vi "MultiPAS-IV.vi"() -> ()   [LabVIEW 2011]
uses:
  <vilib>/Analysis/4window.llb/windowTd.ctl
  sub/QMH/QMH Add Message to Queue (Single Element).vi
  sub/QMH/QMH Add Message to Queue (Array).vi
  <vilib>/measure/maspectr.llb/FFT Spectrum (Mag-Phase) for 1 Chan.vi
  <vilib>/Instr/_visa.llb/VISA Configure Serial Port (Instr).vi
  <vilib>/measure/NI_MAPro.lvlib
  <vilib>/Analysis/NI_AALPro.lvlib
panel:
  out "PAS Save":bool caption="Overtemp"
  in  "Data 2":i32[][](array[numeric])=[[-16374, -7248, 2543, 12030, 20279, 26487, 30037, 30583, 28073, 22744, 15131, 5976, -3818, -13288, -21504, -27663, -31155, -31636, -29064, -23686, -16036, -6862, 2936, 12388, 20571, 26684, 30122, 30546, 27911, 22483, 14793, 5595, -4207, -13644, -21795, -27855, -31232, -31591, -28898, -23423, -15695, -6476, 3323, 12743, 20858, 26873, 30194, 30492, 27744, 22213, 14447, 5207, -4597, -14002, -22082, -28044, -31304, -31540, -28731, -23149, -15348, -6093, 3713, 13101, 21145, 27063, 30265, 30442, 27576, 21943, 14103, 4822, -4984, -14354, -22365, -28230, -31373, -31485, -28556, -22876, -14998, -5702, 4104, 13452, 21428, 27245, 30335, 30388, 27400, 21669, 13754, 4435, -5375, -14705, -22643, -28407, -31436, -31426, -28378, -22598, -14648, -5314, 4497, 13803, 21706, 27423, 30394, 30325, 27221, 21390, 13402, 4045, -5763, -15056, -22921, -28586, -31496, -31361, -28198, -22319, -14297, -4924, 4879, 14151, 21982, 27597, 30451, 30257, 27038, 21107, 13050, 3658, -6149, -15402, -23193, -28754, -31546, -31290, -28010, -22033, -13944, -4536, 5266, 14498, 22252, 27767, 30500, 30184, 26849, 20821, 12696, 3267, -6535, -15748, -23462, -28924, -31596, -31216, -27821, -21748, -13587, -4147, 5653, 14838, 22519, 27930, 30549, 30110, 26658, 20535, 12337, 2878, -6919, -16089, -23727, -29087, -31641, -31137, -27627, -21457, -13229, -3753, 6038, 15181, 22786, 28093, 30591, 30031, 26461, 20243, 11979, 2485, -7303, -16428, -23991, -29244, -31678, -31053, -27426, -21159, -12867, -3360, 6424, 15524, 23043, 28252, 30633, 29946, 26262, 19946, 11617, 2096, -7686, -16764, -24246, -29398, -31712, -30964, -27224, -20862, -12503, -2971, 6803, 15859, 23301, 28401, 30661, 29852, 26058, 19648, 11254, 1703, -8069, -17099, -24500, -29547, -31741, -30870, -27018, -20562, -12138, -2575, 7188, 16192, 23556, 28549, 30689, 29756, 25848, 19348, 10891, 1312, -8448, -17430, -24753, -29691, -31765, -30773, -26806, -20259, -11775, -2186, 7566, 16521, 23801, 28690, 30709, 29656, 25634, 19038, 10523, 919, -8831, -17762, -24997, -29833, -31788, -30672, -26593, -19955, -11409, -1792, 7944, 16850, 24047, 28830, 30724, 29548, 25416, 18729, 10152, 523, -9212, -18092, -25245, -29969, -31805, -30566, -26375, -19647, -11041, -1403, 8319, 17173, 24287, 28963, 30734, 29436, 25192, 18418, 9781, 130, -9587, -18413, -25481, -30101, -31814, -30449, -26150, -19332, -10666, -1007, 8697, 17497, 24524, 29090, 30745, 29325, 24968, 18105, 9408, -263, -9962, -18735, -25718, -30228, -31820, -30334, -25921, -19016, -10296, -618, 9072, 17814, 24756, 29213, 30746, 29202, 24738, 17787, 9036, -657, -10338, -19058, -25951, -30350, -31818, -30214, -25690, -18699, -9922, -224, 9442, 18128, 24984, 29330, 30738, 29078, 24502, 17466, 8658, -1050, -10710, -19371, -26178, -30467, -31814, -30088, -25458, -18382, -9550, 167, 9812, 18440, 25206, 29443, 30732, 28947, 24264, 17143, 8281, -1445, -11083, -19685, -26404, -30581, -31807, -29959, -25221, -18059, -9175, 556, 10178, 18750, 25426, 29548, 30718, 28809, 24018, 16812, 7901, -1842, -11457, -19996, -26624, -30690, -31795, -29824, -24980, -17733, -8799, 950, 10549, 19058, 25643, 29655, 30700, 28673, 23773, 16484, 7523, -2235, -11824, -20304, -26840, -30793, -31772, -29682, -24731, -17402, -8415, 1341, 10916, 19363, 25856, 29755, 30677, 28528, 23522, 16151, 7141, -2626, -12191, -20607, -27051, -30891, -31746, -29536, -24481, -17070, -8035, 1733, 11280, 19664, 26064, 29851, 30648, 28381, 23272, 15818, 6762, -3019, -12555, -20906, -27258, -30984, -31717, -29391, -24226, -16736, -7655, 2128, 11641, 19962, 26270, 29940, 30615, 28229, 23013, 15483, 6376, -3409, -12914, -21204, -27459, -31071, -31684, -29236, -23967, -16398, -7271, 2515, 12005, 20258, 26468, 30024, 30577, 28072, 22753, 15143, 5990, -3802, -13276, -21497, -27660, -31157, -31643, -29076, -23707, -16058, -6886, 2908, 12363, 20550, 26666, 30107, 30536, 27914, 22489, 14805, 5607, -4192, -13633, -21787, -27849, -31230, -31597, -28911, -23438, -15716, -6501, 3298, 12719, 20839, 26858, 30182, 30488, 27744, 22223, 14459, 5225, -4579, -13988, -22071, -28040, -31304, -31549, -28743, -23167, -15368, -6113, 3693, 13076, 21126, 27047, 30255, 30438, 27576, 21950, 14113, 4837, -4971, -14340, -22354, -28224, -31375, -31494, -28570, -22895, -15022, -5725, 4080, 13430, 21408, 27230, 30324, 30384, 27402, 21676, 13766, 4449, -5360, -14694, -22636, -28409, -31440, -31436, -28397, -22617, -14674, -5338, 4467, 13781, 21686, 27408, 30385, 30320, 27224, 21398, 13418, 4062, -5748, -15044, -22913, -28584, -31498, -31368, -28212, -22339, -14321, -4948, 4856, 14131, 21963, 27583, 30440, 30254, 27042, 21118, 13062, 3669, -6137, -15390, -23183, -28751, -31551, -31297, -28024, -22049, -13962, -4556, 5245, 14476, 22235, 27754, 30497, 30186, 26857, 20834, 12710, 3283, -6519, -15733, -23453, -28921, -31600, -31226, -27837, -21765, -13610, -4168, 5628, 14820, 22502, 27918, 30540, 30109, 26664, 20544, 12354, 2891, -6906, -16074, -23719, -29085, -31646, -31148, -27642, -21475, -13251, -3777, 6014, 15160, 22765, 28078, 30583, 30027, 26468, 20251, 11994, 2501, -7292, -16415, -23980, -29242, -31682, -31064, -27443, -21181, -12892, -3386, 6397, 15501, 23026, 28238, 30624, 29944, 26269, 19959, 11633, 2110, -7673, -16753, -24239, -29395, -31719, -30974, -27239, -20882, -12528, -2993, 6782, 15835, 23285, 28390, 30651, 29852, 26063, 19660, 11271, 1720, -8053, -17087, -24493, -29546, -31746, -30880, -27031, -20583, -12163, -2599, 7166, 16173, 23538, 28538, 30684, 29758, 25853, 19356, 10906, 1327, -8433, -17416, -24743, -29688, -31769, -30782, -26821, -20280, -11797, -2208, 7543, 16501, 23786, 28680, 30704, 29656, 25642, 19053, 10540, 936, -8814, -17747, -24989, -29827, -31787, -30678, -26606, -19973, -11430, -1817, 7923, 16829, 24031, 28819, 30721, 29552, 25424, 18746, 10174, 543, -9191, -18072, -25231, -29962, -31802, -30567, -26384, -19660, -11057, -1422, 8302, 17159, 24274, 28952, 30738, 29443, 25205, 18435, 9801, 150, -9568, -18401, -25472, -30095, -31811, -30457, -26163, -19349, -10687, -1031, 8679, 17481, 24511, 29082, 30742, 29327, 24979, 18121, 9431, -241, -9943, -18717, -25707, -30221, -31815, -30337, -25930, -19029, -10312, -631, 9058, 17802, 24745, 29207, 30746, 29209, 24750, 17805, 9057, -634, -10316, -19037, -25937, -30340, -31814, -30217, -25700, -18713, -9939, -240, 9429, 18117, 24976, 29328, 30740, 29088, 24519, 17486, 8682, -1027, -10688, -19352, -26164, -30458, -31810, -30091, -25465, -18390, -9561, 154, 9800, 18433, 25201, 29442, 30735, 28959, 24282, 17165, 8308, -1420, -11063, -19665, -26386, -30570, -31801, -29961, -25227, -18068, -9185, 547, 10171, 18745, 25424, 29552, 30726, 28825, 24038, 16835, 7925, -1815, -11429, -19974, -26608, -30681, -31789, -29826, -24984, -17741, -8807, 938, 10536, 19047, 25636, 29657, 30708, 28685, 23794, 16510, 7550, -2205, -11798, -20280, -26821, -30782, -31766, -29684, -24737, -17411, -8429, 1331, 10906, 19356, 25851, 29758, 30684, 28544, 23546, 16178, 7169, -2598, -12162, -20582, -27035, -30879, -31744, -29540, -24485, -17080, -8048, 1721, 11267, 19655, 26061, 29852, 30654, 28395, 23291, 15843, 6786, -2993, -12527, -20884, -27240, -30974, -31713, -29390, -24230, -16744, -7662, 2115, 11635, 19957, 26268, 29945, 30624, 28246, 23035, 15509, 6406, -3382, -12889, -21180, -27444, -31061, -31677, -29236, -23975, -16408, -7284], [-19329, -1252, 17344, 29341, 30145, 19451, 1353, -17227, -29174, -29920, -19175, -1056, 17506, 29408, 30095, 19300, 1159, -17387, -29238, -29860, -19019, -860, 17671, 29475, 30037, 19143, 960, -17553, -29307, -29809, -18866, -664, 17832, 29545, 29987, 18991, 771, -17707, -29365, -29749, -18707, -466, 17992, 29605, 29926, 18832, 570, -17873, -29434, -29694, -18556, -272, 18151, 29670, 29869, 18676, 375, -18031, -29495, -29633, -18395, -75, 18310, 29729, 29809, 18516, 175, -18194, -29561, -29579, -18238, 120, 18469, 29792, 29750, 18362, -17, -18347, -29617, -29515, -18076, 316, 18629, 29848, 29682, 18197, -218, -18510, -29679, -29456, -17921, 513, 18787, 29910, 29626, 18042, -408, -18664, -29734, -29388, -17757, 709, 18941, 29965, 29560, 17875, -609, -18823, -29791, -29326, -17600, 904, 19095, 30023, 29495, 17717, -802, -18975, -29845, -29260, -17434, 1099, 19251, 30075, 29425, 17551, -1001, -19131, -29901, -29194, -17277, 1296, 19408, 30130, 29359, 17393, -1193, -19284, -29953, -29124, -17112, 1491, 19560, 30184, 29290, 17225, -1392, -19440, -30008, -29056, -16949, 1686, 19713, 30237, 29226, 17069, -1581, -19587, -30054, -28982, -16781, 1883, 19866, 30287, 29151, 16898, -1781, -19742, -30107, -28913, -16616, 2079, 20018, 30337, 29082, 16737, -1973, -19888, -30152, -28838, -16449, 2275, 20167, 30383, 29006, 16564, -2174, -20041, -30200, -28765, -16282, 2471, 20321, 30430, 28934, 16403, -2364, -20187, -30243, -28688, -16113, 2669, 20465, 30470, 28853, 16230, -2568, -20341, -30294, -28618, -15953, 2860, 20615, 30519, 28783, 16070, -2755, -20486, -30335, -28537, -15779, 3057, 20760, 30560, 28700, 15892, -2956, -20637, -30378, -28461, -15613, 3252, 20909, 30605, 28628, 15730, -3145, -20777, -30418, -28377, -15440, 3446, 21054, 30645, 28543, 15557, -3345, -20927, -30460, -28299, -15271, 3643, 21199, 30686, 28465, 15391, -3534, -21066, -30495, -28215, -15100, 3839, 21345, 30722, 28380, 15214, -3734, -21213, -30534, -28134, -14928, 4032, 21487, 30760, 28300, 15044, -3926, -21355, -30570, -28052, -14757, 4225, 21627, 30792, 28209, 14870, -4123, -21501, -30607, -27968, -14586, 4419, 21768, 30832, 28129, 14702, -4314, -21637, -30639, -27880, -14413, 4612, 21907, 30859, 28040, 14521, -4515, -21780, -30675, -27796, -14241, 4804, 22048, 30895, 27953, 14352, -4702, -21919, -30705, -27707, -14064, 4999, 22187, 30922, 27859, 14172, -4900, -22060, -30739, -27620, -13892, 5193, 22326, 30954, 27773, 14003, -5090, -22194, -30765, -27524, -13712, 5386, 22462, 30981, 27679, 13823, -5285, -22333, -30794, -27436, -13538, 5580, 22600, 31013, 27591, 13650, -5476, -22466, -30820, -27343, -13363, 5770, 22732, 31033, 27491, 13468, -5673, -22605, -30848, -27251, -13187, 5964, 22870, 31060, 27401, 13292, -5863, -22736, -30870, -27155, -13010, 6156, 23000, 31079, 27299, 13111, -6058, -22873, -30895, -27060, -12833, 6347, 23134, 31104, 27208, 12936, -6248, -23004, -30918, -26965, -12652, 6536, 23260, 31120, 27106, 12753, -6444, -23136, -30939, -26865, -12472, 6729, 23395, 31148, 27011, 12578, -6634, -23266, -30959, -26766, -12296, 6919, 23523, 31161, 26907, 12392, -6830, -23402, -30982, -26665, -12115, 7109, 23652, 31180, 26809, 12213, -7016, -23524, -30992, -26564, -11932, 7301, 23777, 31195, 26704, 12032, -7210, -23655, -31011, -26464, -11755, 7492, 23907, 31211, 26605, 11855, -7395, -23778, -31024, -26358, -11573, 7680, 24031, 31218, 26494, 11665, -7592, -23908, -31039, -26258, -11392, 7871, 24158, 31237, 26394, 11491, -7775, -24031, -31050, -26153, -11210, 8063, 24281, 31247, 26285, 11302, -7972, -24159, -31062, -26046, -11027, 8250, 24407, 31258, 26180, 11124, -8157, -24276, -31067, -25937, -10841, 8438, 24526, 31265, 26071, 10936, -8347, -24401, -31078, -25829, -10659, 8630, 24649, 31275, 25965, 10755, -8533, -24522, -31087, -25721, -10474, 8816, 24770, 31280, 25853, 10566, -8726, -24641, -31091, -25608, -10290, 9003, 24891, 31287, 25746, 10386, -8910, -24756, -31095, -25498, -10105, 9192, 25008, 31287, 25627, 10196, -9102, -24881, -31101, -25386, -9919, 9381, 25127, 31296, 25521, 10019, -9284, -24994, -31099, -25268, -9732, 9570, 25243, 31293, 25403, 9826, -9476, -25113, -31105, -25157, -9544, 9756, 25359, 31298, 25291, 9645, -9655, -25225, -31099, -25040, -9359, 9942, 25473, 31291, 25167, 9453, -9847, -25341, -31102, -24926, -9173, 10124, 25586, 31294, 25057, 9269, -10029, -25450, -31095, -24809, -8986, 10310, 25696, 31284, 24931, 9078, -10218, -25564, -31094, -24688, -8798, 10497, 25812, 31287, 24819, 8896, -10399, -25673, -31085, -24567, -8608, 10682, 25922, 31278, 24698, 8703, -10587, -25785, -31080, -24448, -8422, 10866, 26033, 31274, 24582, 8522, -10765, -25890, -31067, -24321, -8230, 11050, 26140, 31263, 24455, 8325, -10952, -26001, -31064, -24201, -8040, 11234, 26248, 31255, 24338, 8142, -11132, -26106, -31054, -24079, -7852, 11417, 26353, 31243, 24207, 7948, -11316, -26217, -31041, -23952, -7662, 11601, 26464, 31236, 24089, 7763, -11494, -26315, -31025, -23829, -7471, 11782, 26562, 31217, 23957, 7567, -11682, -26422, -31014, -23702, -7282, 11962, 26667, 31205, 23834, 7383, -11859, -26521, -30998, -23575, -7092, 12144, 26770, 31187, 23704, 7186, -12043, -26626, -30981, -23444, -6900, 12328, 26875, 31176, 23582, 7003, -12218, -26724, -30962, -23316, -6709, 12505, 26971, 31154, 23446, 6805, -12401, -26825, -30946, -23189, -6517, 12687, 27073, 31139, 23322, 6620, -12576, -26919, -30922, -23054, -6323, 12867, 27170, 31114, 23185, 6422, -12760, -27022, -30904, -22923, -6132, 13047, 27272, 31096, 23060, 6237, -12934, -27114, -30879, -22790, -5940, 13222, 27362, 31068, 22921, 6041, -13116, -27212, -30855, -22657, -5748, 13401, 27461, 31048, 22790, 5853, -13289, -27302, -30828, -22522, -5555, 13577, 27549, 31019, 22652, 5652, -13472, -27398, -30806, -22388, -5362, 13753, 27645, 30995, 22521, 5463, -13642, -27487, -30776, -22248, -5169, 13928, 27733, 30963, 22376, 5266, -13823, -27584, -30750, -22113, -4975, 14106, 27828, 30937, 22246, 5082, -13992, -27669, -30717, -21974, -4782, 14280, 27914, 30902, 22101, 4880, -14174, -27760, -30689, -21837, -4588, 14454, 28006, 30875, 21965, 4692, -14340, -27843, -30653, -21693, -4391, 14631, 28092, 30840, 21822, 4494, -14519, -27934, -30620, -21552, -4198, 14805, 28179, 30808, 21688, 4308, -14687, -28015, -30582, -21410, -4004, 14975, 28262, 30770, 21540, 4106, -14861, -28103, -30548, -21268, -3808, 15149, 28349, 30739, 21402, 3916, -15032, -28183, -30512, -21124, -3614, 15319, 28430, 30697, 21255, 3715, -15205, -28267, -30475, -20982, -3421, 15490, 28513, 30664, 21116, 3524, -15376, -28348, -30435, -20837, -3225, 15660, 28592, 30617, 20962, 3327, -15550, -28432, -30397, -20695, -3032, 15829, 28673, 30581, 20820, 3134, -15711, -28506, -30353, -20546, -2837, 15994, 28746, 30530, 20669, 2933, -15887, -28585, -30311, -20400, -2641, 16167, 28828, 30496, 20528, 2745, -16052, -28660, -30264, -20248, -2445, 16335, 28901, 30445, 20376, 2544, -16221, -28737, -30219, -20102, -2250, 16505, 28983, 30406, 20231, 2357, -16381, -28808, -30171, -19950, -2053, 16670, 29053, 30355, 20075, 2154, -16552, -28883, -30127, -19803, -1859, 16835, 29128, 30308, 19930, 1965, -16714, -28952, -30073, -19650, -1663, 17001, 29192, 30255, 19772, 1764, -16881, -29028, -30026, -19496, -1467, 17165, 29268, 30208, 19626, 1572, -17043, -29095, -29977, -19346]]
  out "Filtering":bool caption="Time has Elapsed"
  in  "Switch Filter":bool
  in  "Auto Filter":bool
  out "Elapsed Time (min)":dbl caption="Elapsed Time (s)" format="%#.1g"
  in  "Filter Length (min)":dbl=6.0 caption="Time Target (s)"
  in  "Sample Length (min)":dbl=24.0 caption="Time Target (s)" format="%#.1f"
  out "Time has Elapsed":bool
  in  "Time Target (s)":dbl=1.0
  out "PD Save":bool caption="Overtemp"
  in  "sweep":bool
  in  "All Emit":bool
  in  "Alignment Mode":bool
  in  "660 Emission":bool
  in  "660 Power (mW)":dbl(slide)=100.0 min=0.0 max=100.0 step=1.0 scale=0.0..100.0
  in  "532 Emission":bool
  in  "532 Power (mW)":dbl(slide)=80.0 min=0.0 max=80.0 step=1.0 scale=0.0..80.0
  in  "405 Power (mW)":dbl(slide)=100.0 min=0.0 max=100.0 step=1.0 scale=0.0..100.0
  in  "405 Emission":bool
  out "Overtemp":bool
  in  "Tab Control":T1(tab)=enum."Frequency Sweep"
  in  "Calibration Filepath":path
  in  "Save Cal?":bool=TRUE
  in  "pd id":u32=1
  in  "mic id":u32
  in  "mic cal, scu":dbl=5.41531278804282e-05 format="%#_3e"
  in  "mic cal, scu":dbl=5.59307241877627e-05 format="%#_3e"
  in  "405 Port":refnum<visa-resource-name>="COM70"
  in  "532 Port":refnum<visa-resource-name>="COM26"
  in  "660 Port":refnum<visa-resource-name>="COM69"
  in  "Teensy Port":refnum<visa-resource-name>="COM61"
  in  "Save Mic?":bool
  in  "Mic Time Series File Path":path
  out "error out":errorcluster
  in  "PD Time Series File Path":path
  in  "Save PD?":bool
  in  "Frequency Sweep File Path":path
  in  "Save sweeps?":bool
  in  "Save Abs?":bool
  in  "Abs Time Series File Path":path
  in  "check freqs?":bool=TRUE
  in  "autosweep":bool=TRUE
  in  "set freqs":bool
  out "Frequency Scan":cluster{i32[], "Best Gaussian Fit":dbl[]}[](graph)
  out "Calculated Resonance (Hz)":dbl=1370.0
  in  "Data Start Frequency (Hz)":i32=1355
  in  "Data End Frequency (Hz)":i32=1385
  out "Step No.":i32
  in  "405 F (Hz)":i32=1368
  in  "532 F (Hz)":i32=1372
  in  "660 F (Hz)":i32=1370
  in  "sweep?":bool=TRUE
  in  "660 PD Cal 3":dbl=0.793
  in  "532 PD Cal 3":dbl=0.454
  in  "405 PD Cal 3":dbl=0.237
  out "PD Waveform":waveform(i32)(graph)
  out "PD FFT":cluster{"f0":dbl, "df":dbl, "magnitude":dbl[]}(graph)
  out "pd ts":cluster{dbl, dbl, dbl}(graph)
  in  "Chart Rolling Average Number\n(Transfers to Absorption Data!)":i32=1
  out "mic ts":cluster{dbl, dbl, dbl}(graph)
  out "Mic FFT":cluster{"f0":dbl, "df":dbl, "magnitude":dbl[]}(graph)
  out "Mic Waveform":waveform(i32)(graph)
  in  "calibrate":bool
  in  "GO3 Filepath":path=path "S:/Groups/Smith_G/Photoacoutic Spectroscopy/calibrations/20160810_cal_go3.txt"
  in  "Photodiode Filepath":path=path "S:/Groups/Smith_G/Photoacoutic Spectroscopy/calibrations/20160810_cal_pd.txt"
  in  "Microphone Filepath":path=path "S:/Groups/Smith_G/Photoacoutic Spectroscopy/calibrations/20160810_cal_mic.txt"
  in  "Bkg Start Index":i32=5
  out "aligned data":cluster{"Array":i32[], dbl[]}[](graph)
  out "Calibration":cluster{dbl[], dbl[]}[](graph)
  in  "Bkg End Index":i32=15
  in  "O3 Flow, sccm (80)":dbl=80.0
  in  "660 PD Cal":dbl=0.793
  in  "532 PD Cal":dbl=0.454
  out "532 Slope":dbl
  out "660 Slope":dbl
  out "PAS Cal Coefficient":dbl format="%0.2f"
  in  "GO3 Offset":i32=15
  in  "Cell Calibration, mV/mW":dbl=600000.0
  in  "getbkg":bool
  out "AAE":dbl(graph)
  in  "Bkg Values (mV)":cluster{dbl, dbl, dbl}
  out "Absorption Spectrum":cluster{dbl[], "Best Power Fit":dbl[]}[](graph)
  out "abs ts":cluster{dbl, dbl, dbl}(graph)
  out "Temperatures":T2
  out "Status":string
  in  "Exit":bool
  in  "State Variables":cluster{"CurrentFile":path}
  # "MultiPAS-RGB | AeroSmith Labs (2016)"
  # "Laser Control"
  # "Filter Control"
  # "Communications"
  # "Sound Card Parameters"
  # "Readout"
  # "PD Calibration"
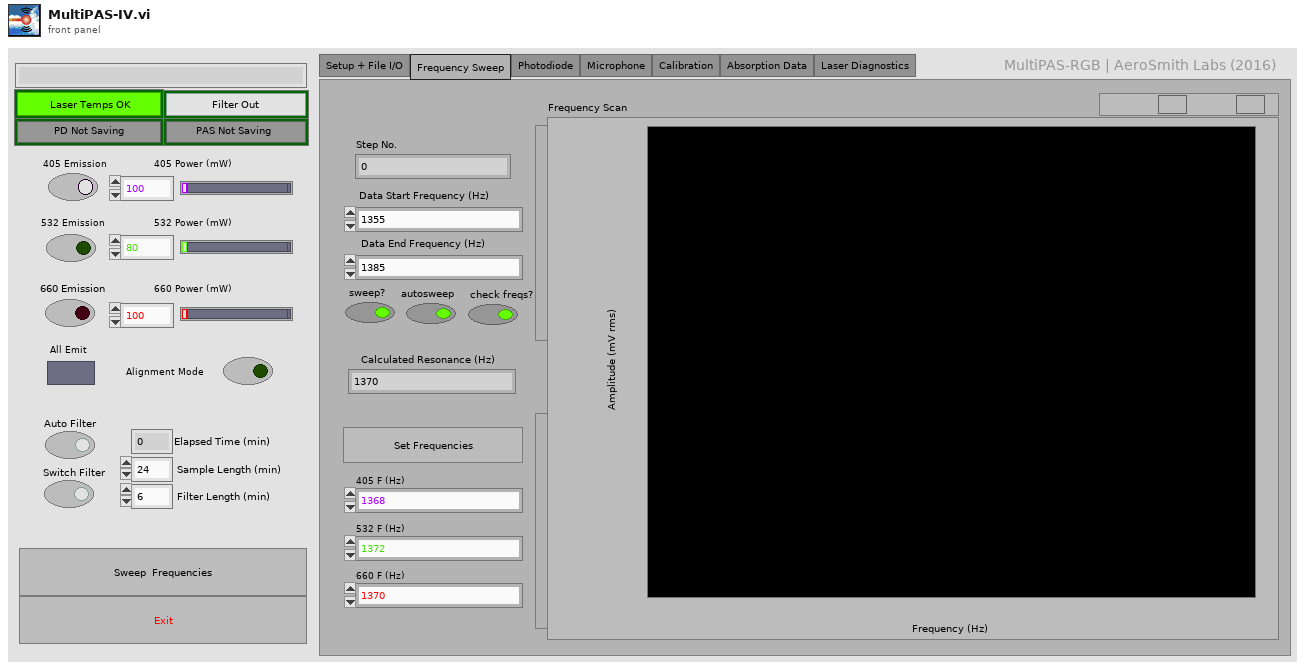
[diagram p1: front panel]
types:
  T1 = enum32{"Setup + File I/O", "Frequency Sweep", "Photodiode", "Microphone", "Calibration", "Absorption Data", "Laser Diagnostics"}
  T2 = cluster{" 405 Temp (C)":dbl, "532 Temp (C)":dbl, "660 Temp (C)":dbl}
  T3 = cluster{"# buffers":i32, "Buffer size":i32, "unit (ms)":enum16{"time (ms)", "Samples"}}
  T4 = typedef "SoundHandle.ctl" = cluster{"DeviceID":u16, "Samples/buf":u32, "Sampl rate":u32, "Bits/sample":u16, "Channels":u8, "Opened":bool}
  T5 = typedef "NI_AALPro.lvlib/windowTd.ctl" = u32
  T6 = cluster{"660 New Array":dbl[], "660 Mean":dbl, "660 SD":dbl}
  T7 = cluster{"532 New Array":dbl[], "532 Mean":dbl, "532 SD":dbl}
  T8 = cluster{"405 New Array":dbl[], "405 Mean":dbl, "405 SD":dbl}
  T9 = cluster{"405 Mean":dbl, "532 Mean":dbl, "660 Mean":dbl}
  T10 = cluster{"Temp (C)":dbl, "Temp (C)":dbl, "Temp (C)":dbl}
  T11 = typedef "LVCursorListTypeDef.ctl" = cluster{"Name":string, "Color":u32, "Style":u8, "Point Style":u8, "Name Visible":bool, "Allow Drag":bool, "Cursor Mode":u32, "Plot":i32, "Index":i32, "Position":cluster{"X":dbl, "Y":dbl}, "X Scale":u32, "Y Scale":u32, "Watch Plots":i32[], "Watch All Plots":bool, "Plot Area":i32, "Label Offset":cluster{"X":dbl, "Y":dbl}}[]
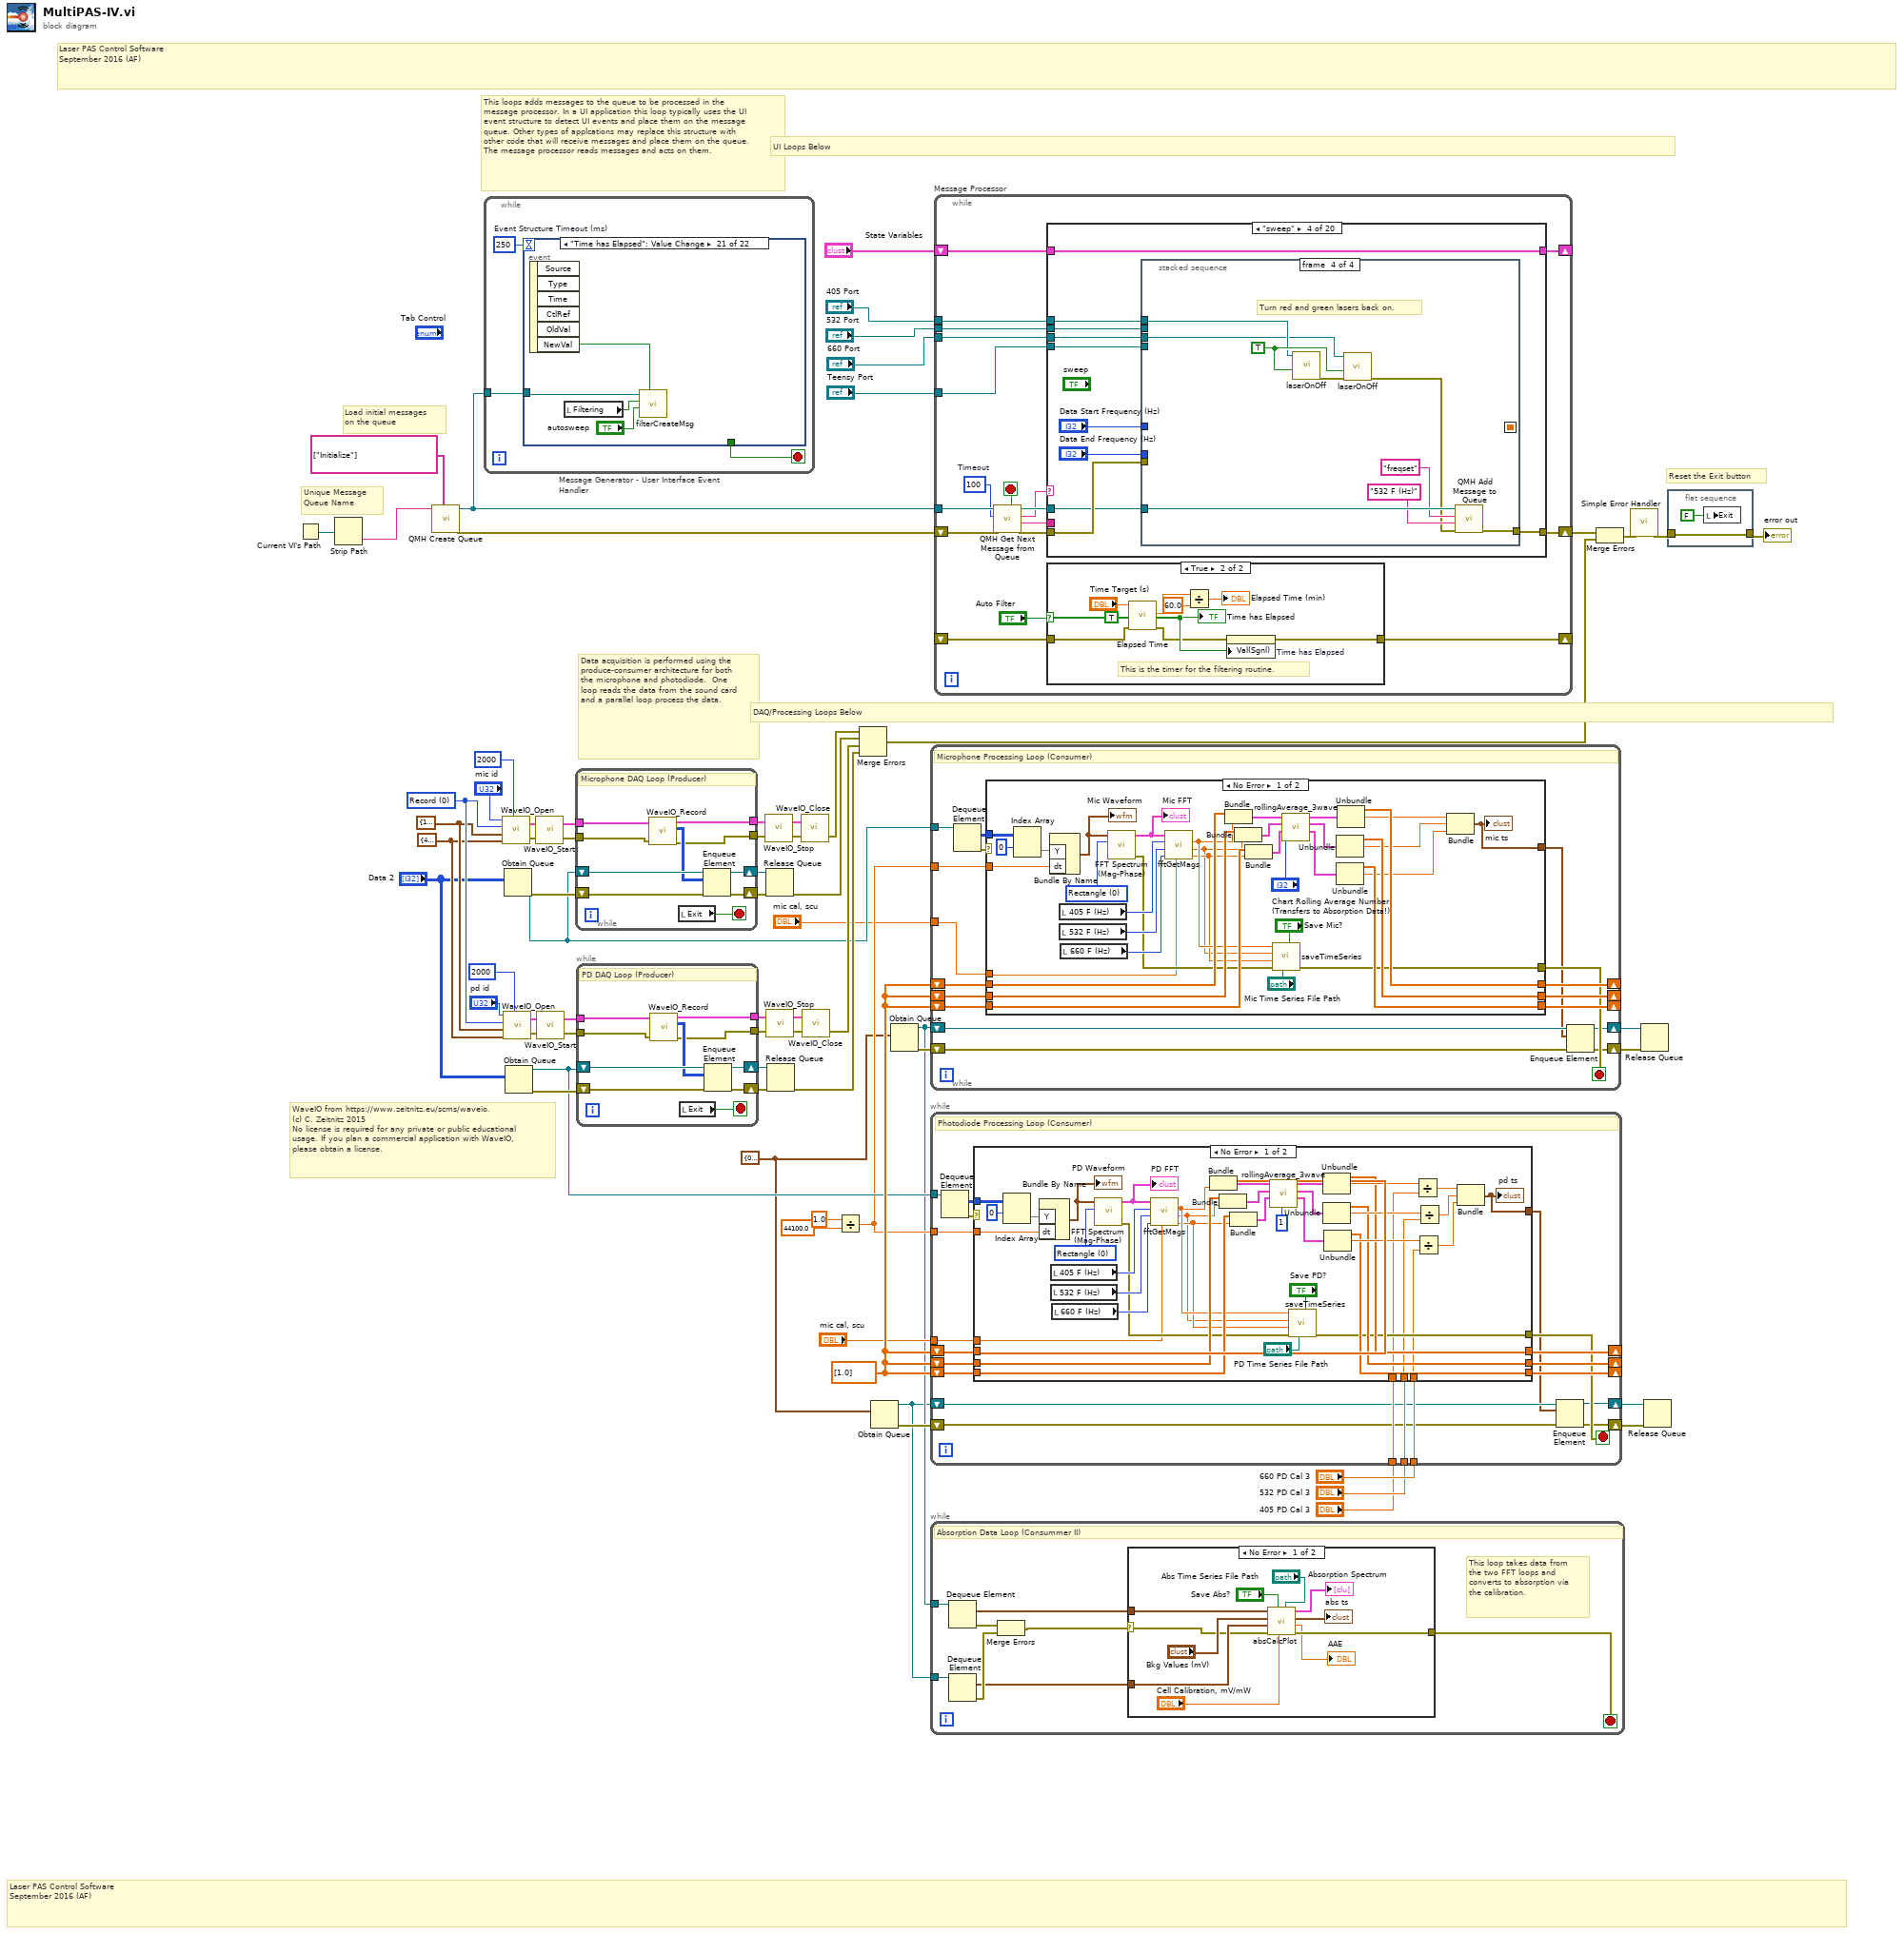
[diagram p0: block diagram]
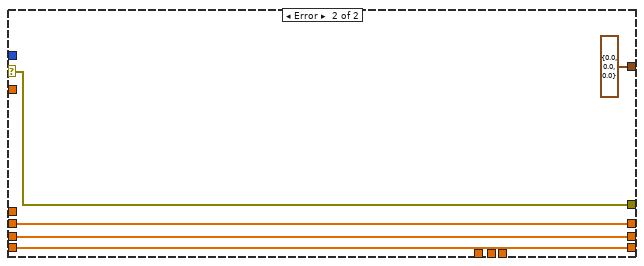
[diagram p3: hidden frame]
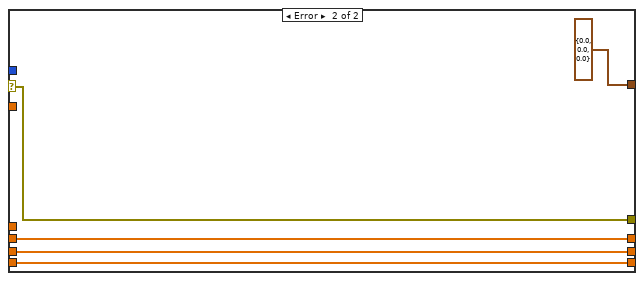
[diagram p4: hidden frame]
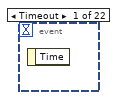
[diagram p5: hidden frame]
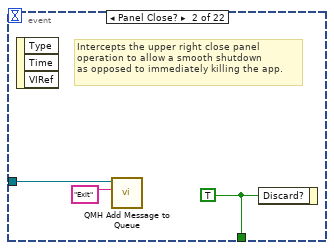
[diagram p6: hidden frame]
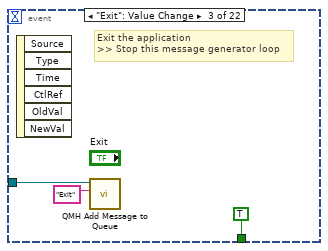
[diagram p7: hidden frame]
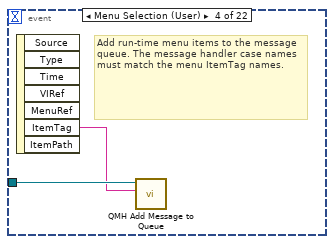
[diagram p8: hidden frame]
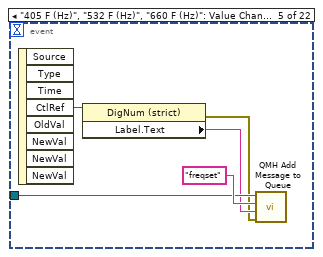
[diagram p9: hidden frame]
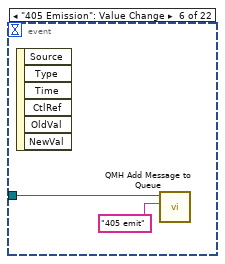
[diagram p10: hidden frame]
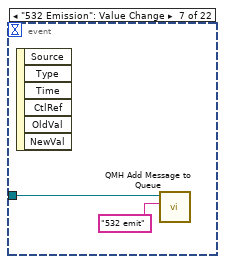
[diagram p11: hidden frame]
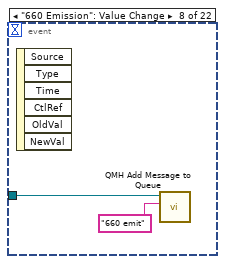
[diagram p12: hidden frame]
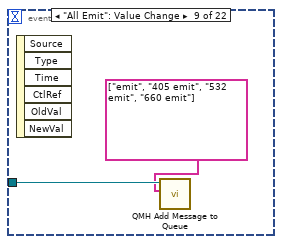
[diagram p13: hidden frame]
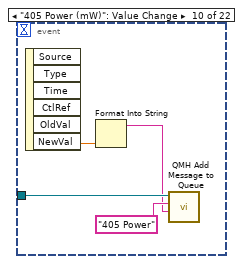
[diagram p14: hidden frame]
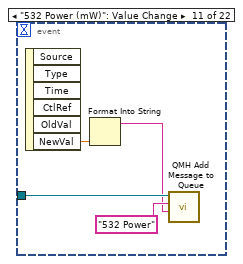
[diagram p15: hidden frame]
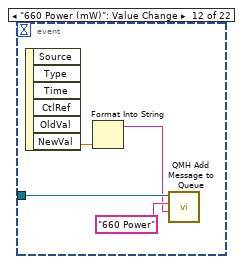
[diagram p16: hidden frame]
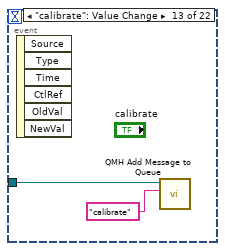
[diagram p17: hidden frame]
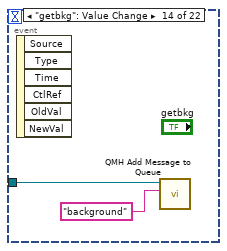
[diagram p18: hidden frame]
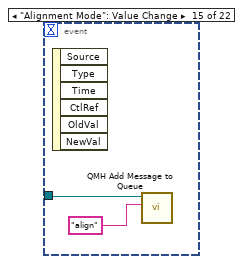
[diagram p19: hidden frame]
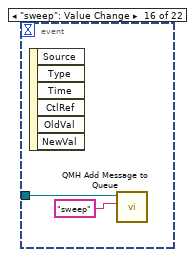
[diagram p20: hidden frame]
diagram:
  w22 = T3 {"# buffers"=10, "Buffer size"=44100, "unit (ms)"=enum."Samples"} ("Buffer")
  w21 = cluster{"Rate":i32, "Bits":i32, "Channels":i32} {"Rate"=44100, "Bits"=24, "Channels"=2} ("Format")
  w1 = cluster{dbl, dbl, dbl} {0.0, 0.0, 0.0}
  w23 = u16 0 items=["Record", "Play", "Loopback", "ASIO input", "ASIO output"] ("Direction (Record)")
  w53 = dbl[] [1.0] ("X")
  # "Laser PAS Control Software\nSeptember 2016 (AF)"
  # "Laser PAS Control Software\nSeptember 2016 (AF)"
  # "Data acquisition is performed using the produce-consumer architecture for both the microphone and photodiode.  One loop reads the data from the sound card and a parallel loop process the data."
  # "WaveIO from https://www.zeitnitz.eu/scms/waveio.\n(c) C. Zeitnitz 2015\nNo license is required for any private or public educational usage. If you plan a commercial application with WaveIO, please obtain a license."
  # "This loops adds messages to the queue to be processed in the message processor. In a UI application this loop typically uses the UI event structure to detect UI events and place them on the message queue. Other types of applcations may replace this structure with other code that will receive messages and place them on the queue.  The message processor reads messages and acts on them."
  # "Reset the Exit button"
  # "Unique Message\nQueue Name"
  # "Load initial messages\non the queue"
  # "DAQ/Processing Loops Below"
  # "UI Loops Below"
  n1 = Current VI's Path() -> (path=w68:path)
  n2 = Strip Path(path=w68) -> (name=w69:string)  [unwired: 1 out]
  n3 = call "QMH Create Queue.vi"("Initial Messages"=string[] ["Initialize"], "Message queue name (unnamed)"=w69) -> ("error out"=w65:errorcluster, "queue out"=w50:refnum<queue>)  [unwired: 8 in]
  n4 = while "Message Generator - User Interface Event Handler" {
    tunnel: w50 -> [w70]
    stop <- w71 stop-if-true
    w72 = 250  # Event Structure Timeout (ms)
    n5 = event shown="[20] \"Time has Elapsed\": Value Change" {
      selector: _ -> [_ _ _ _ _ _ _ _ _ _ _ _ _ _ _ _ _ _ _ _ _ _]
      dyn-events: _ -> [_ _ _ _ _ _ _ _ _ _ _ _ _ _ _ _ _ _ _ _ _ _]
      timeout: w72 -> [_ _ _ _ _ _ _ _ _ _ _ _ _ _ _ _ _ _ _ _ _ _]
      tunnel: [_ w75 TRUE ("Discard?") _ _ _ _ _ _ _ _ _ _ _ _ _ _ _ _ _ _ _] -> w71
      tunnel: w70 -> [_ w74 w77 w80 w84 w86 w88 w90 w93 w96 w100 w104 w106 w108 w110 w113 w117 _ _ w124 w128 w133]
      event Timeout {
        n6 = event-data() -> ()  [unwired: 1 in, 1 out]
      }
      event Panel Close? {
        w75 = TRUE ("Discard?")
        # "Intercepts the upper right close panel\noperation to allow a smooth shutdown\nas opposed to immediately killing the app."
        n7 = event-data() -> ()  [unwired: 1 in, 3 out]
        n8 = call-poly "QMH Add Message to Queue.vi"("Message"="Exit", "queue in"=w74) -> ()  [unwired: 8 in, 2 out]
        n9 = event-data("Discard?"=w75) -> ()  [unwired: 1 in, 1 out]
      }
      event "Exit": Value Change {
        # "Exit the application\n>> Stop this message generator loop"
        n10 = event-data() -> ()  [unwired: 1 in, 6 out]
        n11 = call-poly "QMH Add Message to Queue.vi"("Message"="Exit", "queue in"=w77) -> ()  [unwired: 8 in, 2 out]
      }
      event Menu Selection (User) {
        # "Add run-time menu items to the message\nqueue. The message handler case names must match the menu ItemTag names."
        n12 = event-data() -> ("ItemTag"=w79:string)  [unwired: 1 in, 6 out]
        n13 = call-poly "QMH Add Message to Queue.vi"("Message"=w79, "queue in"=w80) -> ()  [unwired: 8 in, 2 out]
      }
      event "405 F (Hz)", "532 F (Hz)", "660 F (Hz)": Value Change {
        n14 = event-data() -> ("CtlRef"=w83:refnum<vi>)  [unwired: 1 in, 7 out]
        n15 = property class="DigNum (strict)"(reference=w83) -> (error out=w81:errorcluster, "Label.Text"=w82:string)  [unwired: 1 in, 1 out]
        n16 = call-poly "QMH Add Message to Queue.vi"("error in (no error)"=w81, "Parameter"=w82, "Message"="freqset", "queue in"=w84) -> ()  [unwired: 6 in, 2 out]
      }
      event "405 Emission": Value Change {
        n17 = event-data() -> ()  [unwired: 1 in, 6 out]
        n18 = call-poly "QMH Add Message to Queue.vi"("Message"="405 emit", "queue in"=w86) -> ()  [unwired: 8 in, 2 out]
      }
      event "532 Emission": Value Change {
        n19 = event-data() -> ()  [unwired: 1 in, 6 out]
        n20 = call-poly "QMH Add Message to Queue.vi"("Message"="532 emit", "queue in"=w88) -> ()  [unwired: 8 in, 2 out]
      }
      event "660 Emission": Value Change {
        n21 = event-data() -> ()  [unwired: 1 in, 6 out]
        n22 = call-poly "QMH Add Message to Queue.vi"("Message"="660 emit", "queue in"=w90) -> ()  [unwired: 8 in, 2 out]
      }
      event "All Emit": Value Change {
        n23 = event-data() -> ()  [unwired: 1 in, 6 out]
        n24 = call-poly "QMH Add Message to Queue.vi"("Messages"=string[] ["emit", "405 emit", "532 emit", "660 emit"], "queue in"=w93) -> ()  [unwired: 8 in, 2 out]
      }
      event "405 Power (mW)": Value Change {
        n25 = event-data() -> ("NewVal"=w95:dbl)  [unwired: 1 in, 5 out]
        n26 = Format Into String(w95) -> (resulting string=w94:string)  [unwired: 3 in, 1 out]
        n27 = call-poly "QMH Add Message to Queue.vi"("Parameter"=w94, "Message"="405 Power", "queue in"=w96) -> ()  [unwired: 7 in, 2 out]
      }
      event "532 Power (mW)": Value Change {
        n28 = event-data() -> ("NewVal"=w99:dbl)  [unwired: 1 in, 5 out]
        n29 = Format Into String(w99) -> (resulting string=w98:string)  [unwired: 3 in, 1 out]
        n30 = call-poly "QMH Add Message to Queue.vi"("Parameter"=w98, "Message"="532 Power", "queue in"=w100) -> ()  [unwired: 7 in, 2 out]
      }
      event "660 Power (mW)": Value Change {
        n31 = event-data() -> ("NewVal"=w103:dbl)  [unwired: 1 in, 5 out]
        n32 = Format Into String(w103) -> (resulting string=w102:string)  [unwired: 3 in, 1 out]
        n33 = call-poly "QMH Add Message to Queue.vi"("Parameter"=w102, "Message"="660 Power", "queue in"=w104) -> ()  [unwired: 7 in, 2 out]
      }
      event "calibrate": Value Change {
        n34 = event-data() -> ()  [unwired: 1 in, 6 out]
        n35 = call-poly "QMH Add Message to Queue.vi"("Message"="calibrate", "queue in"=w106) -> ()  [unwired: 8 in, 2 out]
      }
      event "getbkg": Value Change {
        n36 = event-data() -> ()  [unwired: 1 in, 6 out]
        n37 = call-poly "QMH Add Message to Queue.vi"("Message"="background", "queue in"=w108) -> ()  [unwired: 8 in, 2 out]
      }
      event "Alignment Mode": Value Change {
        n38 = event-data() -> ()  [unwired: 1 in, 6 out]
        n39 = call-poly "QMH Add Message to Queue.vi"("Message"="align", "queue in"=w110) -> ()  [unwired: 8 in, 2 out]
      }
      event "sweep": Value Change {
        n40 = event-data() -> ()  [unwired: 1 in, 6 out]
        n41 = call-poly "QMH Add Message to Queue.vi"("Message"="sweep", "queue in"=w113) -> ()  [unwired: 8 in, 2 out]
      }
      event "set freqs": Value Change {
        n42 = event-data() -> ()  [unwired: 1 in, 6 out]
        n43 = local read "Calculated Resonance (Hz)"() -> (w116:dbl)
        n44 = Format Into String(w116) -> (resulting string=w115:string, error out=w114:errorcluster)  [unwired: 3 in]
        n45 = call-poly "QMH Add Message to Queue.vi"("error in (no error)"=w114, "Parameter"=w115, "Message"="setfreqs", "queue in"=w117) -> ()  [unwired: 6 in, 2 out]
      }
      event "Save Mic?": Value Change {
        n46 = event-data() -> ("NewVal"=→"PAS Save":bool)  [unwired: 1 in, 5 out]
      }
      event "Save PD?": Value Change {
        n47 = event-data() -> ("NewVal"=→"PD Save":bool)  [unwired: 1 in, 5 out]
      }
      event "Switch Filter": Value Change {
        n48 = event-data() -> ("NewVal"=w123:bool)  [unwired: 1 in, 5 out]
        n49 = local write "Filtering"(w123) -> ()
        n50 = Format Into String(w123) -> (resulting string=w121:string)  [unwired: 3 in, 1 out]
        n51 = call-poly "QMH Add Message to Queue.vi"("Parameter"=w121, "Message"="filterswitch", "queue in"=w124) -> ()  [unwired: 7 in, 2 out]
      }
      event "Time has Elapsed": Value Change {
        n52 = event-data() -> ("NewVal"=w127:bool)  [unwired: 1 in, 5 out]
        n53 = local read "Filtering"() -> (w126:bool)
        n54 = call "filterCreateMsg.vi"("time elapsed?"=w127, "auto sweep (true)"="autosweep", "filtering (true)"=w126, "queue in"=w128) -> ()  [unwired: 6 in, 2 out]
      }
      event "Calculated Resonance (Hz)": Value Change {
        n55 = event-data() -> ("NewVal"=w131:dbl)  [unwired: 1 in, 5 out]
        n56 = Format Into String(w131) -> (resulting string=w129:string, error out=w130:errorcluster)  [unwired: 3 in]
        n57 = call-poly "QMH Add Message to Queue.vi"("error in (no error)"=w130, "Parameter"=w129, "Message"="setfreqs", "queue in"=w133) -> ()  [unwired: 6 in, 2 out]
      }
    }
  }
  n58 = call <userlib>:"WaveIO_Open.vi"("Watchdog timeout (msec) (default=OFF)"=2000, "Format (44kHz, 16Bit, stereo)"=w21, "Buffer Config"=w22, "Direction (Record)"=w23, "idev"="mic id") -> ("error out"=w46:errorcluster, "Sound Handle Out"=w47:T4)  [unwired: 1 in]
  n59 = call <userlib>:"WaveIO_Open.vi"("Watchdog timeout (msec) (default=OFF)"=2000, "Format (44kHz, 16Bit, stereo)"=w21, "Buffer Config"=w22, "Direction (Record)"=w23, "idev"="pd id") -> ("error out"=w32:errorcluster, "Sound Handle Out"=w31:T4)  [unwired: 1 in]
  n60 = Obtain Queue(element data type="Data 2") -> (queue out=w15:refnum<queue>, error out=w54:errorcluster)  [unwired: 4 in, 1 out]
  n61 = Obtain Queue(element data type="Data 2") -> (queue out=w19:refnum<queue>, error out=w28:errorcluster)  [unwired: 4 in, 1 out]
  n62 = call <userlib>:"WaveIO_Start.vi"("error in (no error)"=w46, "Handle"=w47) -> ("error out"=w44:errorcluster, "Handle Out"=w45:T4)
  n63 = call <userlib>:"WaveIO_Start.vi"("error in (no error)"=w32, "Handle"=w31) -> ("error out"=w34:errorcluster, "Handle Out"=w33:T4)
  n64 = while {
    shift-right: [w142] -> w55
    shift-left: w15 -> [w140]
    shift-right: [w143] -> w56
    shift-left: w54 -> [w141]
    tunnel: w45 -> [w138]
    tunnel: w44 -> [w137]
    tunnel: [w135] -> w41
    tunnel: [w134] -> w40
    stop <- w139 stop-if-true
    # "Microphone DAQ Loop (Producer)"
    n65 = call <userlib>:"WaveIO_Record.vi"("Handle"=w138, "error in (no error)"=w137) -> ("Handle Out"=w135:T4, "Data"=w136:i32[][], "error out"=w134:errorcluster)  [unwired: 1 in, 2 out]
    n66 = local read "Exit"() -> (w139:bool)
    n67 = Enqueue Element(queue=w140, element=w136, error in (no error)=w141) -> (queue out=w142:refnum<queue>, error out=w143:errorcluster)  [unwired: 1 in, 1 out]
  }
  n68 = while {
    shift-right: [w152] -> w27
    shift-left: w19 -> [w150]
    shift-right: [w153] -> w26
    shift-left: w28 -> [w151]
    tunnel: w33 -> [w148]
    tunnel: w34 -> [w147]
    tunnel: [w145] -> w37
    tunnel: [w144] -> w38
    stop <- w149 stop-if-true
    # "PD DAQ Loop (Producer)"
    n69 = call <userlib>:"WaveIO_Record.vi"("Handle"=w148, "error in (no error)"=w147) -> ("Handle Out"=w145:T4, "Data"=w146:i32[][], "error out"=w144:errorcluster)  [unwired: 1 in, 2 out]
    n70 = local read "Exit"() -> (w149:bool)
    n71 = Enqueue Element(queue=w150, element=w146, error in (no error)=w151) -> (queue out=w152:refnum<queue>, error out=w153:errorcluster)  [unwired: 1 in, 1 out]
  }
  n72 = call <userlib>:"WaveIO_Stop.vi"("error in (no error)"=w40, "Handle"=w41) -> ("error out"=w42:errorcluster, "Handle Out"=w43:T4)
  n73 = Release Queue(queue=w55, error in (no error)=w56) -> (error out=w52:errorcluster)  [unwired: 1 in, 2 out]
  n74 = call <userlib>:"WaveIO_Stop.vi"("error in (no error)"=w38, "Handle"=w37) -> ("error out"=w36:errorcluster, "Handle Out"=w35:T4)
  n75 = Release Queue(queue=w27, error in (no error)=w26) -> (error out=w25:errorcluster)  [unwired: 1 in, 2 out]
  n76 = call <userlib>:"WaveIO_Close.vi"("error in (no error)"=w42, "Handle"=w43) -> ("error out"=w39:errorcluster)  [unwired: 1 out]
  n77 = call <userlib>:"WaveIO_Close.vi"("error in (no error)"=w36, "Handle"=w35) -> ("error out"=w24:errorcluster)  [unwired: 1 out]
  n78 = Divide(x=1.0, y=44100.0) -> (x/y=w16:dbl)
  n79 = Merge Errors(w39, w52, w24, w25) -> (w51:errorcluster)
  n80 = Obtain Queue(element data type=w1) -> (queue out=w2:refnum<queue>, error out=w6:errorcluster)  [unwired: 4 in, 1 out]
  n81 = Obtain Queue(element data type=w1) -> (queue out=w3:refnum<queue>, error out=w9:errorcluster)  [unwired: 4 in, 1 out]
  n82 = while {
    shift-right: [w171] -> _
    shift-left: w53 -> [w168]
    shift-right: [w170] -> _
    shift-left: w53 -> [w167]
    shift-right: [w169] -> _
    shift-left: w53 -> [w166]
    tunnel: w19 -> [w164]
    tunnel: w16 -> [w163]
    tunnel: "mic cal, scu" -> [w162]
    tunnel: "660 PD Cal 3" -> [w161]
    tunnel: "532 PD Cal 3" -> [w160]
    tunnel: "405 PD Cal 3" -> [w159]
    shift-right: [w156] -> w5
    shift-left: w2 -> [w157]
    shift-right: [w155] -> w4
    shift-left: w6 -> [w158]
    stop <- w165 stop-if-true
    # "Photodiode Processing Loop (Consumer)"
    n83 = Dequeue Element(queue=w164) -> (element=w172:i32[][], error out=w173:errorcluster)  [unwired: 2 in, 2 out]
    n84 = case shown="No Error" w173 {
      selector: w173 -> [_ w216]
      tunnel: w172 -> [w183 _]
      tunnel: w168 -> [w209 w219]
      tunnel: w167 -> [w208 w217]
      tunnel: w166 -> [w207 w218]
      tunnel: [w190 w219] -> w171
      tunnel: [w189 w217] -> w170
      tunnel: [w188 w218] -> w169
      tunnel: [w187 w216] -> w165
      tunnel: w163 -> [w180 _]
      tunnel: w162 -> [w178 _]
      tunnel: w161 -> [w177 _]
      tunnel: w160 -> [w176 _]
      tunnel: w159 -> [w175 _]
      tunnel: [w174 cluster{dbl, dbl, dbl} {0.0, 0.0, 0.0}] -> w154
      frame No Error {
        w211 = T5 0 items=["Rectangle"=0, "Hanning"=1, "Hamming"=2, "Blackman-Harris"=3, "Exact Blackman"=4, "Blackman"=5, "Flat Top"=6, "4 Term B-Harris "=7, "7 Term B-Harris"=8, "Low Sidelobe"=9, "Blackman Nuttall"=11, "Triangle"=30, "Bartlett-Hanning"=31, "Bohman"=32, "Parzen"=33, "Welch"=34, "Kaiser"=60, "Dolph-Chebyshev"=61, "Gaussian"=62] ("window")
        n85 = Index Array(array=w183, index (row)=0) -> (element=w182:i32[])  [unwired: 1 in]
        n86 = Bundle By Name("Y"=w182, "dt"=w180) -> (w181:waveform(i32))  [unwired: 1 in]
        "PD Waveform" <- w181
        n87 = local read "405 F (Hz)"() -> (w214:i32)
        n88 = local read "532 F (Hz)"() -> (w213:i32)
        n89 = local read "660 F (Hz)"() -> (w212:i32)
        n90 = call-poly <vilib>:"FFT Spectrum (Mag-Phase).vi"("window"=w211, "time signal"=w181) -> ("error out"=w203:errorcluster, "magnitude"=w179:cluster{"f0":dbl, "df":dbl, "magnitude":dbl[]})  [unwired: 5 in, 3 out]
        "PD FFT" <- w179
        n91 = call "fftGetMags.vi"("unit cal, scu"=w178, "660 F (Hz)"=w212, "532 F (Hz)"=w213, "405 F (Hz)"=w214, "input cluster"=w179) -> ("mag660 (mV)"=w205:dbl, "mag532 (mV)"=w204:dbl, "mag405 (mV)"=w206:dbl)  [unwired: 4 in]
        n92 = Bundle("X"=w209, "mag405 (mV)"=w206) -> (w210:cluster{"X":dbl[], "mag405 (mV) ":dbl})  [unwired: 1 in]
        n93 = Bundle("X"=w208, "mag532 (mV)"=w204) -> (w201:cluster{"X":dbl[], "mag532 (mV)":dbl})  [unwired: 1 in]
        n94 = Bundle("X"=w207, "mag660 (mV)"=w205) -> (w200:cluster{"X":dbl[], "mag660 (mV)":dbl})  [unwired: 1 in]
        n95 = call "rollingAverage_3wave.vi"("Magnitude Averaging (no. Avgs.)"=1, "660"=w200, "532"=w201, "405"=w210) -> ("660 Data"=w191:T6, "532 Data"=w192:T7, "405 Data"=w193:T8)  [unwired: 5 in]
        n96 = call "saveTimeSeries.vi"("save?"="Save PD?", "file path (dialog if empty)"="PD Time Series File Path", "Error In"=w203, "660nm"=w205, "532nm"=w204, "405nm"=w206) -> ("Error Out"=w187:errorcluster)  [unwired: 5 in]
        n97 = Unbundle(w193) -> ("405 New Array"=w190:dbl[], "405 Mean"=w198:dbl)  [unwired: 1 out]
        n98 = Unbundle(w192) -> ("532 New Array"=w189:dbl[], "532 Mean"=w196:dbl)  [unwired: 1 out]
        n99 = Unbundle(w191) -> ("660 New Array"=w188:dbl[], "660 Mean"=w194:dbl)  [unwired: 1 out]
        n100 = Divide(x=w198, y=w175) -> (x/y=w199:dbl)
        n101 = Divide(x=w194, y=w177) -> (x/y=w195:dbl)
        n102 = Divide(x=w196, y=w176) -> (x/y=w197:dbl)
        n103 = Bundle(w199, w197, w195) -> (w174:cluster{dbl, dbl, dbl})  [unwired: 1 in]
        "pd ts" <- w174
      }
      frame Error {
      }
    }
    n104 = Enqueue Element(queue=w157, element=w154, error in (no error)=w158) -> (queue out=w156:refnum<queue>, error out=w155:errorcluster)  [unwired: 1 in, 1 out]
  }
  n105 = while {
    tunnel: w15 -> [w236]
    shift-right: [w233] -> _
    shift-left: w53 -> [w230]
    shift-right: [w232] -> _
    shift-left: w53 -> [w229]
    shift-right: [w231] -> _
    shift-left: w53 -> [w228]
    tunnel: w16 -> [w226]
    tunnel: "mic cal, scu" -> [w225]
    shift-right: [w223] -> w8
    shift-left: w3 -> [w222]
    shift-right: [w220] -> w7
    shift-left: w9 -> [w224]
    stop <- w227 stop-if-true
    # "Microphone Processing Loop (Consumer)"
    n106 = Dequeue Element(queue=w236) -> (element=w234:i32[][], error out=w235:errorcluster)  [unwired: 2 in, 2 out]
    n107 = case shown="No Error" w235 {
      selector: w235 -> [_ w273]
      tunnel: w234 -> [w246 _]
      tunnel: w230 -> [w266 w276]
      tunnel: w229 -> [w265 w274]
      tunnel: w228 -> [w264 w275]
      tunnel: [w253 w276] -> w233
      tunnel: [w252 w274] -> w232
      tunnel: [w251 w275] -> w231
      tunnel: [w250 w273] -> w227
      tunnel: w226 -> [w243 _]
      tunnel: w225 -> [w241 _]
      tunnel: [w237 T9 {"405 Mean"=0.0, "532 Mean"=0.0, "660 Mean"=0.0}] -> w221
      frame No Error {
        w268 = T5 0 items=["Rectangle"=0, "Hanning"=1, "Hamming"=2, "Blackman-Harris"=3, "Exact Blackman"=4, "Blackman"=5, "Flat Top"=6, "4 Term B-Harris "=7, "7 Term B-Harris"=8, "Low Sidelobe"=9, "Blackman Nuttall"=11, "Triangle"=30, "Bartlett-Hanning"=31, "Bohman"=32, "Parzen"=33, "Welch"=34, "Kaiser"=60, "Dolph-Chebyshev"=61, "Gaussian"=62] ("window")
        n108 = Index Array(array=w246, index (row)=0) -> (element=w245:i32[])  [unwired: 1 in]
        n109 = Bundle By Name("Y"=w245, "dt"=w243) -> (w244:waveform(i32))  [unwired: 1 in]
        "Mic Waveform" <- w244
        n110 = local read "405 F (Hz)"() -> (w271:i32)
        n111 = local read "532 F (Hz)"() -> (w270:i32)
        n112 = local read "660 F (Hz)"() -> (w269:i32)
        n113 = call-poly <vilib>:"FFT Spectrum (Mag-Phase).vi"("window"=w268, "time signal"=w244) -> ("error out"=w260:errorcluster, "magnitude"=w242:cluster{"f0":dbl, "df":dbl, "magnitude":dbl[]})  [unwired: 5 in, 3 out]
        "Mic FFT" <- w242
        n114 = call "fftGetMags.vi"("unit cal, scu"=w241, "660 F (Hz)"=w269, "532 F (Hz)"=w270, "405 F (Hz)"=w271, "input cluster"=w242) -> ("mag660 (mV)"=w262:dbl, "mag532 (mV)"=w261:dbl, "mag405 (mV)"=w263:dbl)  [unwired: 4 in]
        n115 = Bundle("X"=w266, "mag405 (mV)"=w263) -> (w267:cluster{"X":dbl[], "mag405 (mV) ":dbl})  [unwired: 1 in]
        n116 = Bundle("X"=w265, "mag532 (mV)"=w261) -> (w258:cluster{"X":dbl[], "mag532 (mV)":dbl})  [unwired: 1 in]
        n117 = Bundle("X"=w264, "mag660 (mV)"=w262) -> (w257:cluster{"X":dbl[], "mag660 (mV)":dbl})  [unwired: 1 in]
        n118 = call "saveTimeSeries.vi"("save?"="Save Mic?", "file path (dialog if empty)"="Mic Time Series File Path", "Error In"=w260, "660nm"=w262, "532nm"=w261, "405nm"=w263) -> ("Error Out"=w250:errorcluster)  [unwired: 5 in]
        n119 = call "rollingAverage_3wave.vi"("Magnitude Averaging (no. Avgs.)"="Chart Rolling Average Number\n(Transfers to Absorption Data!)", "660"=w257, "532"=w258, "405"=w267) -> ("660 Data"=w254:T6, "532 Data"=w255:T7, "405 Data"=w256:T8)  [unwired: 5 in]
        n120 = Unbundle(w255) -> ("532 New Array"=w252:dbl[], "532 Mean"=w239:dbl)  [unwired: 1 out]
        n121 = Unbundle(w254) -> ("660 New Array"=w251:dbl[], "660 Mean"=w238:dbl)  [unwired: 1 out]
        n122 = Unbundle(w256) -> ("405 New Array"=w253:dbl[], "405 Mean"=w240:dbl)  [unwired: 1 out]
        n123 = Bundle("405 Mean"=w240, "532 Mean"=w239, "660 Mean"=w238) -> (w237:T9)  [unwired: 1 in]
        "mic ts" <- w237
      }
      frame Error {
      }
    }
    n124 = Enqueue Element(queue=w222, element=w221, error in (no error)=w224) -> (queue out=w223:refnum<queue>, error out=w220:errorcluster)  [unwired: 1 in, 1 out]
  }
  n125 = while {
    tunnel: w3 -> [w278]
    tunnel: w2 -> [w277]
    stop <- w283 stop-if-true
    # "This loop takes data from the two FFT loops and converts to absorption via the calibration."
    # "Absorption Data Loop (Consummer II)"
    n126 = Dequeue Element(queue=w278) -> (element=w284:cluster{dbl, dbl, dbl}, error out=w282:errorcluster)  [unwired: 2 in, 2 out]
    n127 = Dequeue Element(queue=w277) -> (element=w279:cluster{dbl, dbl, dbl}, error out=w281:errorcluster)  [unwired: 2 in, 2 out]
    n128 = Merge Errors(w282, w281) -> (w280:errorcluster)
    n129 = case shown="No Error" w280 {
      selector: w280 -> [w288 w296]
      tunnel: w284 -> [w295 _]
      tunnel: [w287 w296] -> w283
      tunnel: w279 -> [w290 _]
      frame No Error {
        n130 = call "absCalcPlot.vi"("file path (dialog if empty)"="Abs Time Series File Path", "Cell Calibration, mV/mW"="Cell Calibration, mV/mW", "save?"="Save Abs?", "Error In"=w288, "PD Values"=w290, "bkg values"="Bkg Values (mV)", "Mic Values"=w295) -> ("Error Out"=w287:errorcluster, "aae"=→"AAE":dbl, "Time Series"=→"abs ts":cluster{dbl, dbl, dbl}, "Spectrum"=→"Absorption Spectrum":cluster{dbl[], "Best Power Fit":dbl[]}[])  [unwired: 1 in]
      }
      frame Error {
      }
    }
  }
  n131 = while "Message Processor" {
    shift-left: w65 -> [w309]
    shift-right: [w301] -> w61
    tunnel: w50 -> [w308]
    shift-left: "State Variables" -> [w314]
    shift-right: [w313] -> _
    tunnel: "405 Port" -> [w305]
    tunnel: "532 Port" -> [w304]
    tunnel: "660 Port" -> [w303]
    tunnel: "Teensy Port" -> [w302]
    shift-right: [w299] -> _
    shift-left: _ -> [w298]
    stop <- w312 stop-if-true
    w306 = 100  # Timeout
    n132 = call "QMH Get Next Message from Queue.vi"("error in (no error)"=w309, "ms timeout (1)"=w306, "queue in"=w308) -> ("error out"=w310:errorcluster, "Next Parameter"=w297:string, "Next Message"=w307:string, "queue out"=w311:refnum<queue>, "Stop QMH"=w312:bool)  [unwired: 3 in]
    n133 = case shown="\"sweep\"" w307 {
      selector: w307 -> [_ w341 _ _ _ _ _ _ _ _ _ _ _ _ _ _ _ _ _ _]
      tunnel: [w337 w342 w355 w365 w421 w444 w476 w483 w489 w495 w501 w509 w516 w523 w543 w550 w574 w593 w622 w633] -> w313
      tunnel: w314 -> [w337 w342 w355 w365 w421 w444 w476 w483 w489 w495 w501 w509 w516 w523 w543 w550 w574 w593 w622 w633]
      tunnel: w311 -> [_ _ _ w358 _ _ _ _ _ _ _ _ _ _ _ _ _ _ w620 w634]
      tunnel: w310 -> [w327 w338 w353 w364 w419 w439 w479 w485 w491 w493 w497 w506 w513 w521 w544 w547 w572 w594 w621 w635]
      tunnel: [w325 w338 w344 w357 w418 w441 w475 w481 w487 w493 w500 w507 w514 w517 w544 w546 w571 w594 w618 w624] -> w301
      tunnel: w305 -> [w331 _ w354 w356 _ _ w478 _ _ _ w502 _ _ w520 _ _ _ _ _ w630]
      tunnel: w304 -> [w330 _ w350 w360 _ _ _ w482 _ _ _ w508 _ w519 _ _ _ _ _ w629]
      tunnel: w303 -> [w329 _ w349 w363 _ _ _ _ w488 _ _ _ w515 w518 _ _ _ _ _ w628]
      tunnel: w302 -> [_ _ w347 w359 w420 w442 _ _ _ _ _ _ _ _ _ w548 w573 _ _ w631]
      tunnel: w297 -> [_ _ _ _ w417 w437 _ _ _ _ w499 w503 w510 _ _ _ w570 _ _ _]
      frame "", "Wait" {
        # "Update the front panel"
        # "Idle Case - this case is called after a Timeout on the Get Next Message from Queue VI, if no new messages are present on the queue. This case can be used for housekeeping tasks such as updating the UI."
        n134 = Get Date/Time String(want seconds? (F)=TRUE) -> (date string=w336:string, time string=w335:string)  [unwired: 2 in]
        n135 = call "laserDiagnose.vi"("error in (no error)"=w327, "660 Port 3"=w329, "532 Port in"=w330, "405 Port"=w331) -> ("error out"=w325:errorcluster, "Temperatures"=→"Temperatures":T10, "Overtemp"=→"Overtemp":bool)  [unwired: 3 in, 2 out]
        n136 = Concatenate Strings(w336, " " ("string"), w335) -> (→"Status":string)
      }
      frame Default {
        # "Call this case if a message is received that is not handled \nby any other case. Typically this is a programming error\nas a result of a typo or unhandled message/missing message handler."
        n137 = Format Into String(format string="DevError: Missing message handler for '%s\" message." ("message"), w341) -> (resulting string=w339:string)  [unwired: 2 in, 1 out]
        n138 = One Button Dialog(message=w339) -> ()  [unwired: 1 in, 1 out]
      }
      frame "Initialize" {
        w351 = u32 115200 ("baud rate (9600)")
        # "Initialize the state variables and user interface\nInitialize serial connections"
        n139 = call-poly "VISA Configure Serial Port"("VISA resource name"=w354, "baud rate (9600)"=w351, "error in (no error)"=w353) -> ("error out"=w352:errorcluster)  [unwired: 11 in, 1 out]
        n140 = call-poly "VISA Configure Serial Port"("VISA resource name"=w350, "baud rate (9600)"=w351, "error in (no error)"=w352) -> ("error out"=w348:errorcluster)  [unwired: 11 in, 1 out]
        n141 = call-poly "VISA Configure Serial Port"("VISA resource name"=w349, "baud rate (9600)"=w351, "error in (no error)"=w348) -> ("error out"=w346:errorcluster)  [unwired: 11 in, 1 out]
        n142 = call-poly "VISA Configure Serial Port"("VISA resource name"=w347, "error in (no error)"=w346) -> ("VISA resource name out"=w345:refnum<visa-resource-name>, "error out"=w343:errorcluster)  [unwired: 12 in]
        n143 = property class="Instr" props=["Baud"](reference=w345, error in=w343) -> (error out=w344:errorcluster)  [unwired: 2 out]
      }
      frame "sweep" {
        # "Perform a frequency sweep and calculate the resonance frequency"
        n144 = stacked-sequence {
          seq-local: [_ w377 _ _] -> [_ _ w403 _]
          tunnel: w364 -> [_ w371 _ _]
          tunnel: "Data End Frequency (Hz)" -> [_ w374 w394 _]
          tunnel: "Data Start Frequency (Hz)" -> [_ w373 w393 _]
          tunnel: w363 -> [w366 _ _ w408]
          tunnel: w360 -> [_ _ _ _]
          tunnel: w359 -> [_ w372 _ _]
          tunnel: w358 -> [_ _ _ w414]
          tunnel: [_ _ _ w410] -> w357
          tunnel: w356 -> [w367 _ _ w409]
          frame #0 {
            w370 = FALSE
            # "Turn red and green lasers off for scan."
            n145 = call "laserOnOff.vi"("Emission (F = OFF)"=w370, "VISA Refnum in"=w367) -> ("error out"=w369:errorcluster)  [unwired: 7 in, 2 out]
            n146 = Wait (ms)(milliseconds to wait=u32 5000) -> ()  [unwired: 1 out]
            n147 = call "laserOnOff.vi"("error in (no error)"=w369, "Emission (F = OFF)"=w370, "VISA Refnum in"=w366) -> ()  [unwired: 6 in, 3 out]
          }
          frame #1 {
            n148 = Subtract(x=w374, y=w373) -> (x-y=w375:i32)
            n149 = for {
              N: w375 -> [_]
              tunnel: [w383] -> w377 mode=indexing
              tunnel: w373 -> [w382]
              tunnel: w374 -> [w381]
              tunnel: w371 -> [_]
              i -> [w380]
              # "Get microphone data."
              # "Listen for N*2000\n seconds"
              n150 = local read "Mic FFT"() -> (w379:cluster{"f0":dbl, "df":dbl, "magnitude":dbl[]})
              n151 = Wait (ms)(milliseconds to wait=u32 2000) -> ()  [unwired: 1 out]
              n152 = Unbundle By Name(w379) -> ("magnitude"=w378:dbl[])
              n153 = call "fftGetMax.vi"("End Frequency (Hz)"=w381, "Start Frequency (Hz)"=w382, "Magnitudes"=w378) -> ("max value"=w383:dbl)  [unwired: 8 in]
              "Step No." <- w380
            }
            n154 = case shown="True" "sweep?" {
              tunnel: w373 -> [_ w390]
              tunnel: w374 -> [_ w389]
              tunnel: w372 -> [_ w388]
              tunnel: [w385 w387] -> _
              tunnel: w371 -> [w385 w386]
              frame False {
              }
              frame True {
                # "Scan laser freq.\nwith Teensy"
                n155 = call "teensySweepFreq.vi"("error in (no error)"=w386, "end f, Hz (1385)"=w389, "start f, Hz (1355)"=w390, "VISA Refnum in"=w388) -> ("error out"=w387:errorcluster)  [unwired: 7 in]
              }
            }
          }
          frame #2 {
            # "Calculate resonance frequency;\ndisplay and save scan."
            n156 = Wait (ms)(milliseconds to wait=u32 5000) -> ()  [unwired: 1 out]
            n157 = To Double Precision Float(number=w394) -> (double precision float=w391:dbl)
            n158 = To Double Precision Float(number=w393) -> (double precision float=w392:dbl)
            n159 = call "resCalc.vi"("Frequency Sweep"=w403, "Start F, Hz (1355)"=w393) -> ("F-res, Hz"=w398:dbl, "Frequency Scan"=w400:cluster{i32[], "Best Gaussian Fit":dbl[]}[])  [unwired: 8 in]
            "Frequency Scan" <- w400
            n160 = In Range and Coerce(upper limit=w391, x=w398, lower limit=w392) -> (In Range?=w397:bool)  [unwired: 1 out]
            n161 = And(x=w397, y="check freqs?") -> (x .and. y?=w395:bool)
            n162 = case shown="True" "Save sweeps?" {
              tunnel: "Frequency Sweep File Path" -> [_ w407]
              tunnel: w400 -> [_ w406]
              tunnel: w398 -> [_ w405]
              frame False {
              }
              frame True {
                n163 = call "saveFreqSweep.vi"("f-res, Hz"=w405, "Frequency Scan"=w406, "file path (dialog if empty)"=w407) -> ()  [unwired: 9 in]
              }
            }
            n164 = case shown="True" w395 {
              tunnel: w398 -> [_ w404]
              frame False {
              }
              frame True {
                n165 = property on="Calculated Resonance (Hz)" class="DigNum (strict)"("Val(Sgnl)"=w404) -> ()  [unwired: 2 in, 2 out]
                "Calculated Resonance (Hz)" <- w404
              }
            }
          }
          frame #3 {
            w415 = TRUE
            # "Turn red and green lasers back on."
            n166 = call "laserOnOff.vi"("Emission (F = OFF)"=w415, "VISA Refnum in"=w409) -> ("error out"=w416:errorcluster)  [unwired: 7 in, 2 out]
            n167 = call "laserOnOff.vi"("error in (no error)"=w416, "Emission (F = OFF)"=w415, "VISA Refnum in"=w408) -> ("error out"=w411:errorcluster)  [unwired: 6 in, 2 out]
            n168 = call-poly "QMH Add Message to Queue.vi"("error in (no error)"=w411, "Parameter"="532 F (Hz)", "Message"="freqset", "queue in"=w414) -> ("error out"=w410:errorcluster)  [unwired: 6 in, 1 out]
          }
        }
      }
      frame "freqset" {
        # "Set the frequency of the Teensy's modulation\nsignal for single laser (if single frequency is changed)."
        # "Set the laser frequency.  Case for \"red\", \"blue\", or \"green\"."
        n169 = case shown="\"532 F (Hz)\"" w417 {
          tunnel: w419 -> [w426 w431 w435]
          tunnel: [w425 w430 w434] -> w418
          tunnel: w420 -> [w422 w427 w432]
          frame "405 F (Hz) ", Default {
            w424 = u16 0 items=["blue", "green", "red"] ("laser")
            n170 = call "freqSet.vi"("error in (no error)"=w426, "laser"=w424, "Freq, Hz (1370)"="405 F (Hz)", "Teensy Port"=w422) -> ("error out"=w425:errorcluster)  [unwired: 6 in, 1 out]
          }
          frame "532 F (Hz)" {
            w429 = u16 1 items=["blue", "green", "red"] ("laser")
            n171 = call "freqSet.vi"("error in (no error)"=w431, "laser"=w429, "Freq, Hz (1370)"="532 F (Hz)", "Teensy Port"=w427) -> ("error out"=w430:errorcluster)  [unwired: 6 in, 1 out]
          }
          frame "660 F (Hz)" {
            w436 = u16 2 items=["blue", "green", "red"] ("laser")
            n172 = call "freqSet.vi"("error in (no error)"=w435, "laser"=w436, "Freq, Hz (1370)"="660 F (Hz)", "Teensy Port"=w432) -> ("error out"=w434:errorcluster)  [unwired: 6 in, 1 out]
          }
        }
      }
      frame "setfreqs" {
        # "Set the frequency of the Teensy's modulation\nsignal for all lasers at once."
        # "Set laser frequencies to resonance frequency calculated in sweep."
        n173 = Scan From String(input string=w437, error in=w439) -> (error out=w438:errorcluster, output 1=w440:dbl)  [unwired: 3 in, 2 out]
        n174 = for {
          N: 3 -> [_]
          tunnel: [w450] -> w441
          tunnel: w438 -> [w449]
          tunnel: w442 -> [w446]
          tunnel: w440 -> [w448]
          i -> [w447]
          n175 = flat-sequence {
            tunnel: w446 -> [w451]
            tunnel: [w451] -> w445
            frame #0 {
              n176 = Wait (ms)(milliseconds to wait=u32 1000) -> ()  [unwired: 1 out]
            }
          }
          n177 = case shown="0" w447 {
            tunnel: [w458 w466 w474] -> w450
            tunnel: w449 -> [w456 w463 w471]
            tunnel: w445 -> [w455 w462 w470]
            tunnel: w448 -> [w453 w459 w467]
            frame 0 {
              w457 = u16 2 items=["blue", "green", "red"] ("laser")
              n178 = To Long Integer(number=w453) -> (32bit integer=w454:i32)
              n179 = local write "660 F (Hz)"(w454) -> ()
              n180 = call "freqSet.vi"("error in (no error)"=w456, "laser"=w457, "Freq, Hz (1370)"=w454, "Teensy Port"=w455) -> ("error out"=w458:errorcluster)  [unwired: 6 in, 1 out]
            }
            frame 1, Default {
              w465 = u16 1 items=["blue", "green", "red"] ("laser")
              n181 = Add(x=w459, y=2.0) -> (x+y=w461:dbl)
              n182 = To Long Integer(number=w461) -> (32bit integer=w460:i32)
              n183 = call "freqSet.vi"("error in (no error)"=w463, "laser"=w465, "Freq, Hz (1370)"=w460, "Teensy Port"=w462) -> ("error out"=w466:errorcluster)  [unwired: 6 in, 1 out]
              n184 = local write "532 F (Hz)"(w460) -> ()
            }
            frame 2 {
              w473 = u16 0 items=["blue", "green", "red"] ("laser")
              n185 = Subtract(x=w467, y=2.0) -> (x-y=w469:dbl)
              n186 = To Long Integer(number=w469) -> (32bit integer=w468:i32)
              n187 = call "freqSet.vi"("error in (no error)"=w471, "laser"=w473, "Freq, Hz (1370)"=w468, "Teensy Port"=w470) -> ("error out"=w474:errorcluster)  [unwired: 6 in, 1 out]
              n188 = local write "405 F (Hz)"(w468) -> ()
            }
          }
        }
      }
      frame "405 emit" {
        # "Turn laser on or off"
        n189 = call "laserOnOff.vi"("error in (no error)"=w479, "Emission (F = OFF)"="405 Emission", "Power, mW (100)"="405 Power (mW)", "VISA Refnum in"=w478) -> ("error out"=w475:errorcluster)  [unwired: 5 in, 2 out]
      }
      frame "532 emit" {
        # "Turn laser on or off"
        n190 = call "laserOnOff.vi"("error in (no error)"=w485, "Emission (F = OFF)"="532 Emission", "Power, mW (100)"="532 Power (mW)", "VISA Refnum in"=w482) -> ("error out"=w481:errorcluster)  [unwired: 5 in, 2 out]
      }
      frame "660 emit" {
        # "Turn laser on or off"
        n191 = call "laserOnOff.vi"("error in (no error)"=w491, "Emission (F = OFF)"="660 Emission", "Power, mW (100)"="660 Power (mW)", "VISA Refnum in"=w488) -> ("error out"=w487:errorcluster)  [unwired: 5 in, 2 out]
      }
      frame "emit" {
        # "Turn on all lasers."
        n192 = local write "405 Emission"("All Emit") -> ()
        n193 = local write "532 Emission"("All Emit") -> ()
        n194 = local write "660 Emission"("All Emit") -> ()
      }
      frame "405 Power" {
        # "Set laser power"
        n195 = Scan From String(input string=w499, error in=w497) -> (error out=w496:errorcluster, output 1=w498:dbl)  [unwired: 3 in, 2 out]
        n196 = call "laserSetPower.vi"("error in (no error)"=w496, "Laser Power (mW)"=w498, "VISA Refnum in"=w502) -> ("error out"=w500:errorcluster)  [unwired: 7 in, 1 out]
      }
      frame "532 Power" {
        n197 = Scan From String(input string=w503, error in=w506) -> (error out=w505:errorcluster, output 1=w504:dbl)  [unwired: 3 in, 2 out]
        n198 = call "laserSetPower.vi"("error in (no error)"=w505, "Laser Power (mW)"=w504, "VISA Refnum in"=w508) -> ("error out"=w507:errorcluster)  [unwired: 7 in, 1 out]
      }
      frame "660 Power" {
        n199 = Scan From String(input string=w510, error in=w513) -> (error out=w512:errorcluster, output 1=w511:dbl)  [unwired: 3 in, 2 out]
        n200 = call "laserSetPower.vi"("error in (no error)"=w512, "Laser Power (mW)"=w511, "VISA Refnum in"=w515) -> ("error out"=w514:errorcluster)  [unwired: 7 in, 1 out]
      }
      frame "align" {
        # "Set power of all lasers to 5 mW for alignment"
        n201 = case shown="True" "Alignment Mode" {
          tunnel: w521 -> [w531 w541]
          tunnel: w520 -> [w530 w540]
          tunnel: w519 -> [w529 w539]
          tunnel: w518 -> [w528 w538]
          tunnel: [w525 w535] -> w517
          frame True {
            w524 = 5.0 ("Laser Power (mW)")
            n202 = call "laserSetPower.vi"("error in (no error)"=w531, "Laser Power (mW)"=w524, "VISA Refnum in"=w530) -> ("error out"=w527:errorcluster)  [unwired: 7 in, 1 out]
            n203 = call "laserSetPower.vi"("error in (no error)"=w527, "Laser Power (mW)"=w524, "VISA Refnum in"=w529) -> ("error out"=w526:errorcluster)  [unwired: 7 in, 1 out]
            n204 = call "laserSetPower.vi"("error in (no error)"=w526, "Laser Power (mW)"=w524, "VISA Refnum in"=w528) -> ("error out"=w525:errorcluster)  [unwired: 7 in, 1 out]
          }
          frame False, Default {
            n205 = local read "405 Power (mW)"() -> (w534:dbl)
            n206 = local read "532 Power (mW)"() -> (w533:dbl)
            n207 = local read "660 Power (mW)"() -> (w532:dbl)
            n208 = call "laserSetPower.vi"("error in (no error)"=w541, "Laser Power (mW)"=w534, "VISA Refnum in"=w540) -> ("error out"=w537:errorcluster)  [unwired: 7 in, 1 out]
            n209 = call "laserSetPower.vi"("error in (no error)"=w537, "Laser Power (mW)"=w533, "VISA Refnum in"=w539) -> ("error out"=w536:errorcluster)  [unwired: 7 in, 1 out]
            n210 = call "laserSetPower.vi"("error in (no error)"=w536, "Laser Power (mW)"=w532, "VISA Refnum in"=w538) -> ("error out"=w535:errorcluster)  [unwired: 7 in, 1 out]
          }
        }
      }
      frame "background" {
        n211 = local read "mic ts"() -> (w542:cluster{dbl, dbl, dbl})
        n212 = local write "Bkg Values (mV)"(w542) -> ()
      }
      frame "filter" {
        n213 = local read "Filtering"() -> (w549:bool)
        n214 = case shown="True" w549 {
          tunnel: w548 -> [w553 w562]
          tunnel: w547 -> [w552 w560]
          tunnel: [w551 w561] -> w546
          frame False {
            n215 = Multiply(x="Filter Length (min)", y=60.0) -> (x*y=w556:dbl)
            n216 = local write "Time Target (s)"(w556) -> ()
            n217 = VISA Write(VISA resource name=w553, write buffer="v.1", error in (no error)=w552) -> (error out=w551:errorcluster)  [unwired: 2 out]
            "Filtering" <- TRUE
          }
          frame True {
            n218 = flat-sequence {
              tunnel: w560 -> [w568]
              tunnel: [w568] -> w559
              frame #0 {
                n219 = local read "mic ts"() -> (w569:cluster{dbl, dbl, dbl})
                n220 = local write "Bkg Values (mV)"(w569) -> ()
              }
            }
            n221 = local write "Filtering"(FALSE) -> ()
            n222 = VISA Write(VISA resource name=w562, write buffer="v.0", error in (no error)=w559) -> (error out=w561:errorcluster)  [unwired: 2 out]
            n223 = Multiply(x="Sample Length (min)", y=60.0) -> (x*y=w564:dbl)
            n224 = local write "Time Target (s)"(w564) -> ()
          }
        }
        n225 = Wait (ms)(milliseconds to wait=u32 500) -> ()  [unwired: 1 out]
      }
      frame "filterswitch" {
        n226 = case shown="\"TRUE\"" w570 {
          tunnel: w573 -> [w577 w582]
          tunnel: w572 -> [w576 w581]
          tunnel: [w575 w580] -> w571
          frame "FALSE", Default {
            n227 = VISA Write(VISA resource name=w577, write buffer="v.0", error in (no error)=w576) -> (error out=w575:errorcluster)  [unwired: 2 out]
          }
          frame "TRUE" {
            n228 = VISA Write(VISA resource name=w582, write buffer="v.1", error in (no error)=w581) -> (error out=w580:errorcluster)  [unwired: 2 out]
          }
        }
      }
      frame "calibrate" {
        n229 = control-ref of="aligned data"() -> (w611:refnum<vi>)
        n230 = call "go3Import.vi"("go3 data"="GO3 Filepath") -> ("flows, sccm"=w613:dbl[][], "[o3], ppb"=w612:dbl[][])  [unwired: 9 in]
        n231 = call "micImport.vi"("mic data"="Microphone Filepath") -> ("mic data"=w603:cluster{dbl[][], dbl[][]})  [unwired: 8 in, 2 out]
        n232 = call "pdImport.vi"("pd data"="Photodiode Filepath") -> ("pd data"=w604:cluster{dbl[][], dbl[][]})  [unwired: 8 in, 2 out]
        n233 = property class="XYGraph (strict)"(reference=w611) -> ("CrsrList"=w610:T11)  [unwired: 1 in, 2 out]
        n234 = call "calNormalize.vi"("532 pd Cal"="532 PD Cal", "660 pd Cal"="660 PD Cal", "pd data"=w604, "mic data"=w603) -> ("660 Normalized"=w607:dbl[], "532 Normalized"=w608:dbl[])  [unwired: 6 in]
        n235 = call "calConvertToND.vi"("O3 Flow, sccm (80)"="O3 Flow, sccm (80)", "flows, sccm"=w613, "[o3], ppb"=w612) -> ("Array"=w598:dbl[])  [unwired: 8 in]
        n236 = call "calDecimateTS.vi"("660 Data"=w607, "532 Data"=w608) -> ("Decimated 660"=w600:dbl[], "Decimated 532"=w599:dbl[])  [unwired: 8 in]
        n237 = call "calSubtractBkg.vi"("bkg end"="Bkg End Index", "bkg start"="Bkg Start Index", "660"=w600, "532"=w599) -> ("660 Substracted"=w591:dbl[], "532 Subtracted"=w592:dbl[])  [unwired: 6 in]
        n238 = call "calSubset.vi"("offset"="GO3 Offset", "CrsrList"=w610, "Decimated 660"=w591, "Decimated 532"=w592, "GO3 Data"=w598) -> ("660 Subset"=w589:dbl[], "532 Subset"=w590:dbl[], "Go3 Subset"=w597:dbl[])  [unwired: 4 in]
        n239 = call "calAlign.vi"("offset"="GO3 Offset", "Decimated 660"=w591, "Decimated 532"=w592, "GO3 Data"=w598) -> ("Aligned Data"=→"aligned data":cluster{"Array":i32[], "Decimated 660":dbl[]}[])  [unwired: 7 in]
        n240 = call "calLinFit.vi"("660 Subset"=w589, "532 Subset"=w590, "Go3 Subset"=w597) -> ("cal coef"=→"PAS Cal Coefficient":dbl, "660 Slope"=w586:dbl, "532 slope"=w587:dbl, "Calibration"=w585:cluster{dbl[], "Best Linear Fit":dbl[]}[])  [unwired: 5 in]
        "Calibration" <- w585
        "532 Slope" <- w587
        "660 Slope" <- w586
        n241 = call "calSave.vi"("O3 flow"="O3 Flow, sccm (80)", "save cal?"="Save Cal?", "m_660"=w586, "m_532"=w587, "Calibration"=w585, "file path (dialog if empty)"="Calibration Filepath") -> ()  [unwired: 6 in]
      }
      frame "Error" {
        (unwired) errorcluster {"status"=FALSE, "code"=0, "source"=""} ("error out")
        # "Proceed to Exit - remove if this is\nnot appropriate for the General Error case"
        # "General Error Case - this case is called if an error is passed using the error cluster below. Typically most new errors should be handed in each individual case and not passed in the rror cluster. If necessary a custom error handler case should be added and called from other cases."
        n242 = call <vilib>:"Simple Error Handler.vi"("error in (no error)"=w621) -> ("error out"=w617:errorcluster)  [unwired: 4 in, 4 out]
        n243 = call-poly "QMH Add Message to Queue.vi"("error in (no error)"=w617, "Message"="Exit", "queue in"=w620) -> ("error out"=w618:errorcluster)  [unwired: 7 in, 1 out]
      }
      frame "Exit" {
        # "Perform cleanup tasks: Close serial connections and clear front panel."
        n244 = call "QMH Destroy Queue.vi"("error in (no error)"=w635, "queue in"=w634) -> ("error out"=w627:errorcluster)  [unwired: 7 in, 2 out]
        n245 = for {
          N: 3 -> [_]
          tunnel: w630 -> [w642]
          tunnel: w629 -> [w640]
          tunnel: w628 -> [w639]
          tunnel: w627 -> [w638]
          tunnel: FALSE -> [w637]
          tunnel: [w636] -> w623
          i -> [w641]
          # "Close laser serial connections."
          n246 = case shown="0, Default" w641 {
            tunnel: [w649 w654 w659] -> w644
            tunnel: [w648 w653 w658] -> w643
            tunnel: w642 -> [w647 _ _]
            tunnel: w640 -> [_ w652 _]
            tunnel: w639 -> [_ _ w656]
            tunnel: w638 -> [w646 w651 w657]
            tunnel: w637 -> [w645 w650 w655]
            frame 0, Default {
              n247 = call "laserOnOff.vi"("error in (no error)"=w646, "Emission (F = OFF)"=w645, "VISA Refnum in"=w647) -> ("error out"=w649:errorcluster, "VISA Refnum out"=w648:refnum<visa-resource-name>)  [unwired: 6 in, 1 out]
              n248 = local write "405 Emission"(w645) -> ()
            }
            frame 1 {
              n249 = call "laserOnOff.vi"("error in (no error)"=w651, "Emission (F = OFF)"=w650, "VISA Refnum in"=w652) -> ("error out"=w654:errorcluster, "VISA Refnum out"=w653:refnum<visa-resource-name>)  [unwired: 6 in, 1 out]
              n250 = local write "532 Emission"(w650) -> ()
            }
            frame 2 {
              n251 = call "laserOnOff.vi"("error in (no error)"=w657, "Emission (F = OFF)"=w655, "VISA Refnum in"=w656) -> ("error out"=w659:errorcluster, "VISA Refnum out"=w658:refnum<visa-resource-name>)  [unwired: 6 in, 1 out]
              n252 = local write "660 Emission"(w655) -> ()
              n253 = local write "All Emit"(w655) -> ()
            }
          }
          n254 = VISA Close(VISA resource name=w643, error in (no error)=w644) -> (error out=w636:errorcluster)
        }
        n255 = local write "Status"("" ("Status")) -> ()
        n256 = VISA Close(VISA resource name=w631, error in (no error)=w623) -> (error out=w624:errorcluster)
      }
    }
    n257 = case shown="True" "Auto Filter" {
      tunnel: [w315 w317] -> w299
      tunnel: w298 -> [w315 w316]
      frame False {
      }
      frame True {
        # "This is the timer for the filtering routine."
        n258 = call "Elapsed Time"("Time Target (s)"="Time Target (s)", "Auto Reset"=TRUE, "error in (no error)"=w316) -> ("Elapsed Time (s)"=w320:dbl, "Time has Elapsed"=w322:bool, "error out"=w321:errorcluster)  [unwired: 9 in, 5 out]
        "Time has Elapsed" <- w322
        n259 = Divide(x=w320, y=60.0) -> (x/y=→"Elapsed Time (min)":dbl)
        n260 = property on="Time has Elapsed" class="Bool (strict)"(error in=w321, "Val(Sgnl)"=w322) -> (error out=w317:errorcluster)  [unwired: 1 in, 1 out]
      }
    }
  }
  n261 = Merge Errors(w61, w51) -> (w60:errorcluster)
  n262 = call <vilib>:"Simple Error Handler.vi"("error in (no error)"=w60) -> ("error out"=w59:errorcluster)  [unwired: 4 in, 4 out]
  n263 = Release Queue(queue=w8, error in (no error)=w7) -> ()  [unwired: 1 in, 3 out]
  n264 = Release Queue(queue=w5, error in (no error)=w4) -> ()  [unwired: 1 in, 3 out]
  n265 = flat-sequence {
    tunnel: w59 -> [w660]
    tunnel: [w660] -> w58
    frame #0 {
      n266 = local write "Exit"(FALSE) -> ()
    }
  }
  "error out" <- w58
